vi "SCMP - Main Program.vi"() -> ()   [LabVIEW 2014]
doc: "Goodrich Exposure Range: .05microseconds to 798.9ms\n\nLow Gain (110e-/ADU)\nHigh Gain (6.5 e-/ADU)\n\nGA1280J Trigger Modes\n0 : Internally triggered; Internally timed\n1 : Externally triggered; Internally timed\n2 : Externally triggered; Externally timed\n3 : Externally gated; Internally timed\n\nFor list of camera commands\nsee Appendix A in the manual\n\n\nUse this template to build a standard state machine design pattern. Each state executes code and determines which state to transition to. Contrast this design pattern with the User Interface Event Handler pattern, in which code executes in response to user actions. Contrast this design pattern also with the Queued Message Handler pattern, in which each message handling code can queue zero or more new messages.\nNote: This template does not contain the most recent programming guidelines recommended by National Instruments. For a complete, project-based implementation of the Standard State Machine pattern, use the Create Project dialog box instead of this template."
uses:
  Controls/Main Program States.ctl
  <vilib>/Utility/error.llb/DialogType.ctl
  Controls/SCD - Calibration Optics Filter Wheel.ctl
  Controls/SCD - EDT - Emission Line Filter Wheel.ctl
  COMP/CoMP-S Controls/Emission Line Filter Wheel.ctl
  COMP/CoMP-S Controls/Polarization Optics Filter Wheel.ctl
  Controls/Global demo.vi
  C:/Users/mhutar/Documents/miro/lv_workdir github/SCMP/LabVIEW/COMP/Watlow EZ-ZONE/Public/Watbus.dll
  LabVIEW/COMP/Watlow EZ-ZONE/Public/Watbus.dll
  Controls/SCD - FITS Cluster.ctl
  AISAS/Controls/focus.ctl
  AISAS/Controls/Diffuser.ctl
  AISAS/Mech/AISAS Mech.lvclass
  Controls/peripherals.ctl
  Controls/Cbk Data type.ctl
  Controls/Cookbook.ctl
  Controls/beaning.ctl
  LabVIEW/Camera/Andor Neo Info.ctl
  PI/PI Control.ctl
panel:
  out "Instrument":string
  out "Main Loop":bool
  out "Log Loop":bool
  out "Program":bool
  out "Version":string
  in  "AOI Width 2":i64=2560
  in  "AOI Height 2":i64=2160
  in  "Observer":string="Observer"
  in  "Comment":string="Test"
  out "Latest Actions":string="\r"
  out "cbk name":string="automated_find_focus_656.cbk"
  out "Last Error":errorcluster={"status"=TRUE, "code"=0, "source"=""}
  in  "Tab Control":T1(tab)
  in  "PI cam3 (mm)":T2 min=0.1 max=27.0 step=0.1 format="%.1f"
  in  "PI cam2 (mm)":T2 min=0.1 max=31.0 step=0.1 format="%.1f"
  in  "Calibration Optics":T3
  in  "Occulter size":dbl format="%.2f"
  in  "Focus":T4 min=15.0 max=155.0 format="%.2f"
  in  "Andover Filter Wheel":T5
  in  "Calibration Wheel":T6
  in  "Binning":T7
  in  "Save Data to FITS? (F)":bool
  out "Histogram Graph":T8(graph)
  in  "Snap Images":bool
  in  "Live Preview (Andor)":bool
  out "Image":u16[][](graph)
  in  "Exposure (s)":dbl=0.02 min=1e-05 max=10.0 step=0.001 format="%_3p"
  out "Timestamp":timestamp=timestamp(3507746192.5616717 s since 1904-01-01)
  in  "PI cam1 (mm)":T2 min=0.1 max=29.0 step=0.1 format="%.1f"
  out "Snapshot FITS File Path":path
  in  "Emission Line Filters":T9
  in  "Set Filter Wheels":bool
  out "Mean ADU":u32=7788 format="%.1f"
  out "FITS Header":T10={"Wavelength (nm)"=530.15, "Exposure (s)"=0.05, "Tuning Delay (ms)"=1000.0, "Beam Type (-1/1)"=1.0, "Tuning Voltages"=[1.111, 2.222, 3.333, 4.444], "Observer"="observer", "Light Shapping Diffuser"=enum."In Beam", "Comment"="", "Data Type"=9, "Mod Cycles"=0, "SCD Calibration Optics"=enum."1 - Polarizer @0, I+Q", "SCD Emission Line Filter"=enum."1-557.6nm", "Cookbook"="", "COMP-S Calibration Wheel"=enum."Dark", "COMP-S Andover Filter Wheel"=enum."530.3nm/HWB 0.34nm (Fe XIV)", "FOV Rotation (deg)"=66.0, "Objective Lens Position (mm)"=0.0, "Occulter size"=0.0, "Time End"=timestamp(3382374145.421875 s since 1904-01-01), "Acc Exposure (s)"=0.0, "Time Stamp Array"=[], "Camera Serial Number"=[], "Camera Temp"=[], "Camera PI (mm)"=[], "Time Start"=timestamp(3382374145.421875 s since 1904-01-01), "Peripherals"={"ILX controler"=FALSE, "Zone temperatures"=FALSE, "Andor"=FALSE, "Andor 2"=FALSE, "PI Stage"=FALSE, "AISAS mechanisms"=FALSE, "AISAS Mech.lvclass"=refnum, "Zone temp ref"=variant}} {"Camera PI (mm)" format="%_3g"; "Acc Exposure (s)" format="%^.3g"; "Occulter size" format="%.2f"; "Objective Lens Position (mm)" min=15.0 max=155.0 format="%.2f"; "FOV Rotation (deg)" format="%.1f"; "Data Type" items=["LIVE", "DARK", "FLAT", "CALI", "OBSE", "ABSO", "AURE", "TARG", "OBJE", "HOLE", "OREX", "THRO", "CHIP"]; "Exposure (s)" format="%^.3g"; "Wavelength (nm)" format="%_6g"}
  out "Image Sharpness":dbl format="%.2f"
  in  "Diffuser":T11=enum."In Beam"
  in  "Rotation [deg]":dbl format="%.1f"
  in  "Move AISAS Mechanisms":bool
  in  "Motors":bool=TRUE
  out "Andor Neo":T13[](array[typedef]) {"Exposure (s)" format="%^.3g"; "Time at Synch" format="%<%H:%M:%S>T"; "Interframe Time" format="%#_3g"; "Frame Readout Time" format="%_3g"; "Row Readout Time" format="%_3g"}
  in  "Save Data to FITS?":bool=TRUE
  out "Cookbook":T15=[{"Data Type"=enum."SET EXPOSURE", "Arg 1"=200.0, "Arg 2"=999.0, "Arg 3"=path "C:/CoMP-S_Observer_cbks_rcps/mhutar/exposure-200ms.rcp", "Comments"=""}, {"Data Type"=enum."ACQUIRE DATA", "Arg 1"=1.0, "Arg 2"=1.0, "Arg 3"=path "C:/CoMP-S_Observer_cbks_rcps/mhutar/scan_530_3.rcp", "Comments"=""}]
  out "FITS Path from Last Recipe Acquiring Data":path
  in  "Load Cookbook":bool
  in  "Run Cookbook":bool
  out "# of Recipes":i16=2
  out "Selected Cookbook":path
  out "Recipe Files":string[](array[string])
  in  "FPS":dbl=10.0 min=0.1 max=49.0 step=1.0 format="%.1g"
  out "Continually Read Log File":string="20160903-07:42:55 Live Preview Images\n20160903-07:44:38 Program Terminated\n20160903-07:45:16 Program Started\n20160903-07:45:18 Snap Single Image\n20160903-07:45:27 Live Preview Images\n20160903-07:46:17 Calibration & Filter wheel position:\t8\t5\n20160903-07:46:35 Live Preview Images\n20160903-07:50:39 Live Preview Images\n20160903-07:51:54 Camera Moved to Positon:-18.00\n20160903-07:51:55 Snap Single Image\n20160903-07:52:37 Loaded Cookbook\tfind_focus_656.cbk\n20160903-07:53:52 Run Cookbook\tfind_focus_656.cbk\n20160903-07:53:52 Recipe#0-exposure-20ms.rcp\n20160903-07:53:52 Recipe#1-fw-656.rcp\n20160903-07:53:54 Recipe#2-cal-open.rcp\n20160903-07:53:56 Recipe#3-move-absolute-neg19.rcp\n20160903-07:53:56 Recipe#4-take_656_focus_image.rcp\n20160903-07:54:02 Recipe#5-move-relative-neg0pt25.rcp\n20160903-07:55:56 Program Started\n20160903-07:56:02 Camera Moved to Positon:-18.00\n20160903-07:56:03 Snap Single Image\n20160903-07:56:35 Camera Moved to Positon:-19.00\n20160903-07:56:37 Snap Single Image\n20160903-07:56:58 Camera Moved to Positon:-20.00\n20160903-07:57:02 Snap Single Image\n20160903-07:57:20 Camera Moved to Positon:-21.00\n20160903-07:57:23 Snap Single Image\n20160903-07:57:36 Camera Moved to Positon:-22.00\n20160903-07:57:37 Snap Single Image\n20160903-07:57:53 Camera Moved to Positon:-25.00\n20160903-07:57:57 Snap Single Image\n20160903-07:58:13 Camera Moved to Positon:-30.00\n20160903-07:58:17 Snap Single Image\n20160903-07:58:43 Camera Moved to Positon:-18.00\n20160903-07:58:44 Snap Single Image\n20160903-07:58:58 Camera Moved to Positon:-17.00\n20160903-07:59:00 Snap Single Image\n20160903-08:00:39 Calibration & Filter wheel position:\t7\t6\n20160903-08:00:48 Snap Single Image\n20160903-08:01:42 Camera Moved to Positon:-65.00\n20160903-08:01:47 Snap Single Image\n20160903-08:02:07 Camera Moved to Positon:-70.00\n20160903-08:02:10 Snap Single Image\n20160903-08:02:51 Camera Moved to Positon:-75.00\n20160903-08:02:53 Snap Single Image\n20160903-08:03:25 Calibration & Filter wheel position:\t7\t7\n20160903-08:03:37 Snap Single Image\n20160903-08:03:55 Camera Moved to Positon:-76.00\n20160903-08:04:01 Snap Single Image\n20160903-08:04:13 Camera Moved to Positon:-77.00\n20160903-08:04:14 Snap Single Image\n20160903-08:04:24 Camera Moved to Positon:-78.00\n20160903-08:04:26 Snap Single Image\n20160903-08:04:38 Camera Moved to Positon:-79.00\n20160903-08:04:39 Snap Single Image\n20160903-08:04:50 Camera Moved to Positon:-83.00\n20160903-08:04:52 Snap Single Image\n20160903-08:05:10 Camera Moved to Positon:-73.00\n20160903-08:05:11 Snap Single Image\n20160903-08:05:22 Camera Moved to Positon:-71.00\n20160903-08:05:24 Snap Single Image\n20160903-08:05:34 Camera Moved to Positon:-69.00\n20160903-08:05:35 Snap Single Image\n20160903-08:05:47 Camera Moved to Positon:-67.00\n20160903-08:05:48 Snap Single Image\n20160903-08:06:13 Calibration & Filter wheel position:\t7\t8\n20160903-08:07:06 Snap Single Image\n20160903-08:07:17 Camera Moved to Positon:-69.00\n20160903-08:07:18 Snap Single Image\n20160903-08:07:28 Camera Moved to Positon:-71.00\n20160903-08:07:30 Snap Single Image\n20160903-08:07:40 Camera Moved to Positon:-73.00\n20160903-08:07:43 Snap Single Image\n20160903-08:07:53 Camera Moved to Positon:-75.00\n20160903-08:07:55 Snap Single Image\n20160903-08:08:04 Camera Moved to Positon:-77.00\n20160903-08:08:06 Snap Single Image\n20160903-08:08:17 Camera Moved to Positon:-79.00\n20160903-08:08:28 Snap Single Image\n20160903-08:08:43 Camera Moved to Positon:-81.00\n20160903-08:08:46 Snap Single Image\n20160903-08:09:05 Calibration & Filter wheel position:\t7\t9\n20160903-08:09:48 Camera Moved to Positon:-100.00\n20160903-08:09:50 Snap Single Image\n20160903-08:10:09 Snap Single Image\n20160903-08:10:26 Camera Moved to Positon:-100.00\n20160903-08:10:35 Camera Moved to Positon:-100.00\n20160903-08:10:37 Snap Single Image\n20160903-08:10:54 Camera Moved to Positon:-100.00\n20160903-08:10:59 Program Terminated\n20160903-08:12:25 Program Started\n20160903-08:12:33 Camera Moved to Positon:-100.00\n20160903-08:12:38 Program Terminated\n20160903-08:13:25 Program Started\n20160903-08:13:30 Camera Moved to Positon:-100.00\n20160903-08:13:37 Program Terminated\n20160903-08:14:12 Program Started\n20160903-08:14:19 Camera Moved to Positon:-100.00\n20160903-08:14:22 Snap Single Image\n20160903-08:14:37 Calibration & Filter wheel position:\t7\t9\n20160903-08:14:45 Snap Single Image\n20160903-08:14:56 Camera Moved to Positon:-105.00\n20160903-08:14:57 Snap Single Image\n20160903-08:15:10 Camera Moved to Positon:-110.00\n20160903-08:15:11 Snap Single Image\n20160903-08:15:23 Camera Moved to Positon:-115.00\n20160903-08:15:27 Snap Single Image\n20160903-08:15:39 Camera Moved to Positon:-120.00\n20160903-08:15:40 Snap Single Image\n20160903-08:15:59 Snap Single Image\n20160903-08:16:10 Camera Moved to Positon:-115.00\n20160903-08:16:11 Snap Single Image\n20160903-08:16:21 Camera Moved to Positon:-110.00\n20160903-08:16:22 Snap Single Image\n20160903-08:16:33 Camera Moved to Positon:-105.00\n20160903-08:16:36 Snap Single Image\n20160903-08:16:49 Camera Moved to Positon:-100.00\n20160903-08:16:51 Snap Single Image\n20160903-08:17:03 Camera Moved to Positon:-95.00\n20160903-08:17:05 Snap Single Image\n20160903-08:17:16 Camera Moved to Positon:-90.00\n20160903-08:17:18 Snap Single Image\n20160903-08:17:46 Camera Moved to Positon:-85.00\n20160903-08:17:49 Snap Single Image\n20160903-08:18:00 Camera Moved to Positon:-80.00\n20160903-08:18:02 Snap Single Image\n20160903-08:18:40 Calibration & Filter wheel position:\t7\t4\n20160903-08:18:59 Camera Moved to Positon:-20.00\n20160903-08:19:11 Snap Single Image\n20160903-08:19:23 Camera Moved to Positon:-18.00\n20160903-08:19:25 Snap Single Image\n20160903-08:19:38 Camera Moved to Positon:-22.00\n20160903-08:19:39 Snap Single Image\n20160903-08:19:51 Camera Moved to Positon:-24.00\n20160903-08:19:52 Snap Single Image\n20160903-08:20:04 Calibration & Filter wheel position:\t7\t3\n20160903-08:20:11 Snap Single Image\n20160903-08:20:22 Camera Moved to Positon:-18.00\n20160903-08:20:24 Snap Single Image\n20160903-08:20:39 Camera Moved to Positon:-16.00\n20160903-08:20:40 Snap Single Image\n20160903-08:20:53 Camera Moved to Positon:-14.00\n20160903-08:20:56 Snap Single Image\n20160903-08:21:06 Camera Moved to Positon:-12.00\n20160903-08:21:07 Snap Single Image\n20160903-08:21:16 Camera Moved to Positon:-10.00\n20160903-08:21:24 Snap Single Image\n20160903-08:21:34 Camera Moved to Positon: -8.00\n20160903-08:21:36 Snap Single Image\n20160903-08:22:12 Camera Moved to Positon: -6.00\n20160903-08:22:21 Snap Single Image\n20160903-08:23:09 Calibration & Filter wheel position:\t7\t1\n20160903-08:23:17 Snap Single Image\n20160903-08:23:27 Camera Moved to Positon: -4.00\n20160903-08:23:29 Snap Single Image\n20160903-08:23:37 Camera Moved to Positon: -2.00\n20160903-08:23:38 Snap Single Image\n20160903-08:23:47 Camera Moved to Positon:  0.00\n20160903-08:23:50 Snap Single Image\n20160903-08:26:00 Camera Moved to Positon:-18.00\n20160903-08:26:44 Program Started\n20160903-08:26:59 Camera Moved to Positon:-18.00\n20160903-08:27:05 Loaded Cookbook\tfind_focus_656.cbk\n20160903-08:27:12 Run Cookbook\tfind_focus_656.cbk\n20160903-08:27:12 Recipe#0-exposure-20ms.rcp\n20160903-08:27:12 Recipe#1-fw-656.rcp\n20160903-08:27:14 Recipe#2-cal-open.rcp\n20160903-08:27:16 Recipe#3-take_656_focus_image.rcp\n20160903-08:29:11 Camera Moved to Positon:-19.00\n20160903-08:29:17 Run Cookbook\tfind_focus_656.cbk\n20160903-08:29:17 Recipe#0-exposure-20ms.rcp\n20160903-08:29:17 Recipe#1-fw-656.rcp\n20160903-08:29:19 Recipe#2-cal-open.rcp\n20160903-08:29:21 Recipe#3-take_656_focus_image.rcp\n20160903-08:29:59 Camera Moved to Positon:-20.00\n20160903-08:30:03 Run Cookbook\tfind_focus_656.cbk\n20160903-08:30:03 Recipe#0-exposure-20ms.rcp\n20160903-08:30:03 Recipe#1-fw-656.rcp\n20160903-08:30:05 Recipe#2-cal-open.rcp\n20160903-08:30:07 Recipe#3-take_656_focus_image.rcp\n20160903-08:30:28 Camera Moved to Positon:-21.00\n20160903-08:30:32 Run Cookbook\tfind_focus_656.cbk\n20160903-08:30:32 Recipe#0-exposure-20ms.rcp\n20160903-08:30:32 Recipe#1-fw-656.rcp\n20160903-08:30:34 Recipe#2-cal-open.rcp\n20160903-08:30:36 Recipe#3-take_656_focus_image.rcp\n20160903-08:31:03 Camera Moved to Positon:-22.00\n20160903-08:31:06 Run Cookbook\tfind_focus_656.cbk\n20160903-08:31:06 Recipe#0-exposure-20ms.rcp\n20160903-08:31:06 Recipe#1-fw-656.rcp\n20160903-08:31:08 Recipe#2-cal-open.rcp\n20160903-08:31:10 Recipe#3-take_656_focus_image.rcp\n20160903-08:31:33 Camera Moved to Positon:-23.00\n20160903-08:31:38 Run Cookbook\tfind_focus_656.cbk\n20160903-08:31:38 Recipe#0-exposure-20ms.rcp\n20160903-08:31:38 Recipe#1-fw-656.rcp\n20160903-08:31:40 Recipe#2-cal-open.rcp\n20160903-08:31:42 Recipe#3-take_656_focus_image.rcp\n20160903-08:32:05 Camera Moved to Positon:-24.00\n20160903-08:32:08 Run Cookbook\tfind_focus_656.cbk\n20160903-08:32:08 Recipe#0-exposure-20ms.rcp\n20160903-08:32:08 Recipe#1-fw-656.rcp\n20160903-08:32:10 Recipe#2-cal-open.rcp\n20160903-08:32:12 Recipe#3-take_656_focus_image.rcp\n20160903-08:32:35 Camera Moved to Positon:-25.00\n20160903-08:32:40 Run Cookbook\tfind_focus_656.cbk\n20160903-08:32:40 Recipe#0-exposure-20ms.rcp\n20160903-08:32:40 Recipe#1-fw-656.rcp\n20160903-08:32:42 Recipe#2-cal-open.rcp\n20160903-08:32:44 Recipe#3-take_656_focus_image.rcp\n20160903-08:33:03 Camera Moved to Positon:-26.00\n20160903-08:33:07 Run Cookbook\tfind_focus_656.cbk\n20160903-08:33:07 Recipe#0-exposure-20ms.rcp\n20160903-08:33:07 Recipe#1-fw-656.rcp\n20160903-08:33:09 Recipe#2-cal-open.rcp\n20160903-08:33:11 Recipe#3-take_656_focus_image.rcp\n20160903-08:33:32 Camera Moved to Positon:-27.00\n20160903-08:33:34 Run Cookbook\tfind_focus_656.cbk\n20160903-08:33:34 Recipe#0-exposure-20ms.rcp\n20160903-08:33:34 Recipe#1-fw-656.rcp\n20160903-08:33:36 Recipe#2-cal-open.rcp\n20160903-08:33:38 Recipe#3-take_656_focus_image.rcp\n20160903-08:34:01 Camera Moved to Positon:-28.00\n20160903-08:34:05 Run Cookbook\tfind_focus_656.cbk\n20160903-08:34:05 Recipe#0-exposure-20ms.rcp\n20160903-08:34:05 Recipe#1-fw-656.rcp\n20160903-08:34:07 Recipe#2-cal-open.rcp\n20160903-08:34:09 Recipe#3-take_656_focus_image.rcp\n20160903-08:36:44 Camera Moved to Positon:-85.00\n20160903-08:36:51 Loaded Cookbook\tfind_focus_1083.cbk\n20160903-08:37:11 Loaded Cookbook\tfind_focus_1083.cbk\n20160903-08:37:20 Run Cookbook\tfind_focus_1083.cbk\n20160903-08:37:20 Recipe#0-exposure-120ms.rcp\n20160903-08:37:20 Recipe#1-fw-1083.rcp\n20160903-08:37:22 Recipe#2-cal-open.rcp\n20160903-08:37:23 Recipe#3-take_1083_focus_image.rcp\n20160903-08:38:05 Camera Moved to Positon:-86.00\n20160903-08:38:11 Run Cookbook\tfind_focus_1083.cbk\n20160903-08:38:11 Recipe#0-exposure-120ms.rcp\n20160903-08:38:11 Recipe#1-fw-1083.rcp\n20160903-08:38:13 Recipe#2-cal-open.rcp\n20160903-08:38:15 Recipe#3-take_1083_focus_image.rcp\n20160903-08:38:39 Camera Moved to Positon:-87.00\n20160903-08:38:43 Run Cookbook\tfind_focus_1083.cbk\n20160903-08:38:43 Recipe#0-exposure-120ms.rcp\n20160903-08:38:43 Recipe#1-fw-1083.rcp\n20160903-08:38:45 Recipe#2-cal-open.rcp\n20160903-08:38:47 Recipe#3-take_1083_focus_image.rcp\n20160903-08:39:05 Camera Moved to Positon:-88.00\n20160903-08:39:09 Run Cookbook\tfind_focus_1083.cbk\n20160903-08:39:10 Recipe#0-exposure-120ms.rcp\n20160903-08:39:10 Recipe#1-fw-1083.rcp\n20160903-08:39:12 Recipe#2-cal-open.rcp\n20160903-08:39:13 Recipe#3-take_1083_focus_image.rcp\n20160903-08:43:45 Snap Single Image\n20160903-08:43:56 Run Cookbook\tfind_focus_1083.cbk\n20160903-08:43:56 Recipe#0-exposure-120ms.rcp\n20160903-08:43:56 Recipe#1-fw-1083.rcp\n20160903-08:43:58 Recipe#2-cal-open.rcp\n20160903-08:44:00 Recipe#3-take_1083_focus_image.rcp\n20160903-08:44:24 Camera Moved to Positon:-90.00\n20160903-08:44:32 Camera Moved to Positon:-89.00\n20160903-08:44:36 Run Cookbook\tfind_focus_1083.cbk\n20160903-08:44:36 Recipe#0-exposure-120ms.rcp\n20160903-08:44:36 Recipe#1-fw-1083.rcp\n20160903-08:44:38 Recipe#2-cal-open.rcp\n20160903-08:44:40 Recipe#3-take_1083_focus_image.rcp\n20160903-08:45:03 Camera Moved to Positon:-90.00\n20160903-08:45:11 Run Cookbook\tfind_focus_1083.cbk\n20160903-08:45:12 Recipe#0-exposure-120ms.rcp\n20160903-08:45:12 Recipe#1-fw-1083.rcp\n20160903-08:45:14 Recipe#2-cal-open.rcp\n20160903-08:45:15 Recipe#3-take_1083_focus_image.rcp\n20160903-08:45:38 Camera Moved to Positon:-91.00\n20160903-08:45:41 Run Cookbook\tfind_focus_1083.cbk\n20160903-08:45:41 Recipe#0-exposure-120ms.rcp\n20160903-08:45:42 Recipe#1-fw-1083.rcp\n20160903-08:45:43 Recipe#2-cal-open.rcp\n20160903-08:45:45 Recipe#3-take_1083_focus_image.rcp\n20160903-08:46:07 Camera Moved to Positon:-92.00\n20160903-08:46:12 Run Cookbook\tfind_focus_1083.cbk\n20160903-08:46:12 Recipe#0-exposure-120ms.rcp\n20160903-08:46:12 Recipe#1-fw-1083.rcp\n20160903-08:46:14 Recipe#2-cal-open.rcp\n20160903-08:46:16 Recipe#3-take_1083_focus_image.rcp\n20160903-08:46:53 Camera Moved to Positon:-93.00\n20160903-08:46:56 Run Cookbook\tfind_focus_1083.cbk\n20160903-08:46:56 Recipe#0-exposure-120ms.rcp\n20160903-08:46:56 Recipe#1-fw-1083.rcp\n20160903-08:46:58 Recipe#2-cal-open.rcp\n20160903-08:47:00 Recipe#3-take_1083_focus_image.rcp\n20160903-08:48:13 Calibration & Filter wheel position:\t7\t3\n20160903-08:51:11 Camera Moved to Positon:-10.00\n20160903-08:51:19 Camera Moved to Positon: -5.00\n20160903-08:51:20 Live Preview Images\n20160903-08:51:43 Loaded Cookbook\tfind_focus_589.cbk\n20160903-08:52:08 Loaded Cookbook\tfocus-656.cbk\n20160903-08:52:09 Run Cookbook\tfocus-656.cbk\n20160903-08:52:09 Recipe#0-fw-656.rcp\n20160903-08:52:11 Recipe#1-cal-clear.rcp\n20160903-08:52:13 Recipe#2-exposure-200ms.rcp\n20160903-08:52:13 Recipe#3-focus-656.rcp\n20160903-08:52:24 Program Started\n20160903-08:52:33 Loaded Cookbook\tfocus-656.cbk\n20160903-08:52:40 Camera Moved to Positon: -5.00\n20160903-08:52:46 Loaded Cookbook\tfind_focus_589.cbk\n20160903-08:52:48 Run Cookbook\tfind_focus_589.cbk\n20160903-08:52:48 Recipe#0-exposure-20ms.rcp\n20160903-08:52:48 Recipe#1-fw-589.rcp\n20160903-08:52:50 Recipe#2-cal-open.rcp\n20160903-08:52:52 Recipe#3-take_589_focus_image.rcp\n20160903-08:54:55 Run Cookbook\tfind_focus_589.cbk\n20160903-08:54:55 Recipe#0-exposure-20ms.rcp\n20160903-08:54:56 Recipe#1-fw-589.rcp\n20160903-08:54:57 Recipe#2-cal-open.rcp\n20160903-08:54:59 Recipe#3-take_589_focus_image.rcp\n20160903-08:55:19 Live Preview Images\n20160903-08:56:01 Camera Moved to Positon: -6.00\n20160903-08:56:04 Run Cookbook\tfind_focus_589.cbk\n20160903-08:56:04 Recipe#0-exposure-20ms.rcp\n20160903-08:56:04 Recipe#1-fw-589.rcp\n20160903-08:56:06 Recipe#2-cal-open.rcp\n20160903-08:56:08 Recipe#3-take_589_focus_image.rcp\n20160903-08:56:40 Camera Moved to Positon: -7.00\n20160903-08:58:30 Run Cookbook\tfind_focus_589.cbk\n20160903-08:58:30 Recipe#0-exposure-20ms.rcp\n20160903-08:58:30 Recipe#1-fw-589.rcp\n20160903-08:58:32 Recipe#2-cal-open.rcp\n20160903-08:58:34 Recipe#3-take_589_focus_image.rcp\n20160903-08:59:22 Camera Moved to Positon: -8.00\n20160903-09:14:18 Program Terminated\n20160903-09:40:55 Program Started\n20160903-09:44:03 Loaded Cookbook\tautomated_find_focus_656.cbk\n20160903-09:44:43 Loaded Cookbook\tautomated_find_focus_656.cbk\n20160903-09:44:57 Run Cookbook\tautomated_find_focus_656.cbk\n20160903-09:44:57 Recipe#0-exposure-20ms.rcp\n20160903-09:44:57 Recipe#1-fw-656.rcp\n20160903-09:44:59 Recipe#2-cal-open.rcp\n20160903-09:45:01 Recipe#3-move-absolute-neg15.rcp\n20160903-09:45:02 Recipe#4-take_656_focus_image.rcp\n20160903-09:45:16 Recipe#5-move-relative-neg0pt25.rcp\n20160903-09:45:17 Recipe#6-take_656_focus_image.rcp\n20160903-09:45:31 Recipe#7-move-relative-neg0pt25.rcp\n20160903-09:45:32 Recipe#8-take_656_focus_image.rcp\n20160903-09:45:46 Recipe#9-move-relative-neg0pt25.rcp\n20160903-09:45:47 Recipe#10-take_656_focus_image.rcp\n20160903-09:46:01 Recipe#11-move-relative-neg0pt25.rcp\n20160903-09:46:02 Recipe#12-take_656_focus_image.rcp\n20160903-09:46:17 Recipe#13-move-relative-neg0pt25.rcp\n20160903-09:46:18 Recipe#14-take_656_focus_image.rcp\n20160903-09:46:32 Recipe#15-move-relative-neg0pt25.rcp\n20160903-09:46:33 Recipe#16-take_656_focus_image.rcp\n20160903-09:46:47 Recipe#17-move-relative-neg0pt25.rcp\n20160903-09:46:48 Recipe#18-take_656_focus_image.rcp\n20160903-09:47:02 Recipe#19-move-relative-neg0pt25.rcp\n20160903-09:47:03 Recipe#20-take_656_focus_image.rcp\n20160903-09:47:17 Recipe#21-move-relative-neg0pt25.rcp\n20160903-09:47:17 Recipe#22-take_656_focus_image.rcp\n20160903-09:47:32 Recipe#23-move-relative-neg0pt25.rcp\n20160903-09:47:32 Recipe#24-take_656_focus_image.rcp\n20160903-09:47:46 Recipe#25-move-relative-neg0pt25.rcp\n20160903-09:47:47 Recipe#26-take_656_focus_image.rcp\n20160903-09:48:02 Recipe#27-move-relative-neg0pt25.rcp\n20160903-09:48:03 Recipe#28-take_656_focus_image.rcp\n20160903-09:48:17 Recipe#29-move-relative-neg0pt25.rcp\n20160903-09:48:17 Recipe#30-take_656_focus_image.rcp\n20160903-09:48:32 Recipe#31-move-relative-neg0pt25.rcp\n20160903-09:48:33 Recipe#32-take_656_focus_image.rcp\n20160903-09:48:49 Recipe#33-move-relative-neg0pt25.rcp\n20160903-09:48:49 Recipe#34-take_656_focus_image.rcp\n20160903-09:49:05 Recipe#35-move-relative-neg0pt25.rcp\n20160903-09:49:06 Recipe#36-take_656_focus_image.rcp\n20160903-09:49:23 Recipe#37-move-relative-neg0pt25.rcp\n20160903-09:49:24 Recipe#38-take_656_focus_image.rcp\n20160903-09:49:41 Recipe#39-move-relative-neg0pt25.rcp\n20160903-09:49:42 Recipe#40-take_656_focus_image.rcp\n20160903-09:50:01 Recipe#41-move-relative-neg0pt25.rcp\n20160903-09:50:01 Recipe#42-take_656_focus_image.rcp\n20160903-09:50:20 Recipe#43-move-relative-neg0pt25.rcp\n20160903-09:50:21 Recipe#44-take_656_focus_image.rcp\n20160903-09:54:36 Loaded Cookbook\tautomated_find_focus_656.cbk\n20160903-09:54:47 Loaded Cookbook\tautomated_find_focus_656.cbk\n20160903-09:55:40 Loaded Cookbook\tautomated_find_focus_656.cbk\n20160903-09:55:54 Run Cookbook\tautomated_find_focus_656.cbk\n20160903-09:55:54 Recipe#0-exposure-40ms.rcp\n20160903-09:55:54 Recipe#1-fw-656.rcp\n20160903-09:55:56 Recipe#2-cal-open.rcp\n20160903-09:55:58 Recipe#3-move-absolute-neg15.rcp\n20160903-09:55:59 Recipe#4-take_656_focus_image.rcp\n20160903-09:56:06 Recipe#5-move-relative-neg0pt5.rcp\n20160903-09:56:07 Recipe#6-take_656_focus_image.rcp\n20160903-09:56:14 Recipe#7-move-relative-neg0pt5.rcp\n20160903-09:56:15 Recipe#8-take_656_focus_image.rcp\n20160903-09:56:22 Recipe#9-move-relative-neg0pt5.rcp\n20160903-09:56:22 Recipe#10-take_656_focus_image.rcp\n20160903-09:56:29 Recipe#11-move-relative-neg0pt5.rcp\n20160903-09:56:30 Recipe#12-take_656_focus_image.rcp\n20160903-09:56:37 Recipe#13-move-relative-neg0pt5.rcp\n20160903-09:56:38 Recipe#14-take_656_focus_image.rcp\n20160903-09:56:45 Recipe#15-move-relative-neg0pt5.rcp\n20160903-09:56:45 Recipe#16-take_656_focus_image.rcp\n20160903-09:56:52 Recipe#17-move-relative-neg0pt5.rcp\n20160903-09:56:53 Recipe#18-take_656_focus_image.rcp\n20160903-09:57:00 Recipe#19-move-relative-neg0pt5.rcp\n20160903-09:57:01 Recipe#20-take_656_focus_image.rcp\n20160903-09:57:08 Recipe#21-move-relative-neg0pt5.rcp\n20160903-09:57:09 Recipe#22-take_656_focus_image.rcp\n20160903-09:57:16 Recipe#23-move-relative-neg0pt5.rcp\n20160903-09:57:16 Recipe#24-take_656_focus_image.rcp\n20160903-09:57:23 Recipe#25-move-relative-neg0pt5.rcp\n20160903-09:57:24 Recipe#26-take_656_focus_image.rcp\n20160903-09:57:31 Recipe#27-move-relative-neg0pt5.rcp\n20160903-09:57:32 Recipe#28-take_656_focus_image.rcp\n20160903-09:57:39 Recipe#29-move-relative-neg0pt5.rcp\n20160903-09:57:40 Recipe#30-take_656_focus_image.rcp\n20160903-09:57:47 Recipe#31-move-relative-neg0pt5.rcp\n20160903-09:57:48 Recipe#32-take_656_focus_image.rcp\n20160903-09:57:55 Recipe#33-move-relative-neg0pt5.rcp\n20160903-09:57:56 Recipe#34-take_656_focus_image.rcp\n20160903-09:58:03 Recipe#35-move-relative-neg0pt5.rcp\n20160903-09:58:03 Recipe#36-take_656_focus_image.rcp\n20160903-09:58:10 Recipe#37-move-relative-neg0pt5.rcp\n20160903-09:58:11 Recipe#38-take_656_focus_image.rcp\n20160903-09:58:18 Recipe#39-move-relative-neg0pt5.rcp\n20160903-09:58:19 Recipe#40-take_656_focus_image.rcp\n20160903-09:58:26 Recipe#41-move-relative-neg0pt5.rcp\n20160903-09:58:27 Recipe#42-take_656_focus_image.rcp\n20160903-09:58:34 Recipe#43-move-relative-neg0pt5.rcp\n20160903-09:58:35 Recipe#44-take_656_focus_image.rcp\n20160903-10:46:33 Program Terminated\n20160903-12:25:32 Program Started\n20160903-12:26:22 Program Terminated\n20160903-12:45:45 Program Started\n20160903-12:45:56 Program Terminated\n20160903-12:49:12 Program Started\n20160903-12:49:15 Loaded Cookbook\tautomated_find_focus_656.cbk\n20160903-12:49:24 Run Cookbook\tautomated_find_focus_656.cbk\n20160903-12:49:25 Recipe#0-exposure-40ms.rcp\n20160903-12:49:25 Recipe#1-fw-656.rcp\n20160903-12:49:26 Recipe#2-cal-open.rcp\n20160903-12:49:28 Recipe#3-move-absolute-neg15.rcp\n20160903-12:49:29 Recipe#4-take_656_focus_image.rcp\n20160903-12:49:32 Recipe#5-move-relative-neg0pt5.rcp\n20160903-12:49:33 Recipe#6-take_656_focus_image.rcp\n20160903-12:49:36 Recipe#7-move-relative-neg0pt5.rcp\n20160903-12:49:36 Recipe#8-take_656_focus_image.rcp\n20160903-12:49:39 Recipe#9-move-relative-neg0pt5.rcp\n20160903-12:49:40 Recipe#10-take_656_focus_image.rcp\n20160903-12:49:43 Recipe#11-move-relative-neg0pt5.rcp\n20160903-12:49:43 Recipe#12-take_656_focus_image.rcp\n20160903-12:49:46 Recipe#13-move-relative-neg0pt5.rcp\n20160903-12:49:47 Recipe#14-take_656_focus_image.rcp\n20160903-12:49:49 Recipe#15-move-relative-neg0pt5.rcp\n20160903-12:49:50 Recipe#16-take_656_focus_image.rcp\n20160903-12:49:53 Recipe#17-move-relative-neg0pt5.rcp\n20160903-12:49:53 Recipe#18-take_656_focus_image.rcp\n20160903-12:49:56 Recipe#19-move-relative-neg0pt5.rcp\n20160903-12:49:57 Recipe#20-take_656_focus_image.rcp\n20160903-12:49:59 Recipe#21-move-relative-neg0pt5.rcp\n20160903-12:50:00 Recipe#22-take_656_focus_image.rcp\n20160903-12:50:03 Recipe#23-move-relative-neg0pt5.rcp\n20160903-12:50:04 Recipe#24-take_656_focus_image.rcp\n20160903-12:50:06 Recipe#25-move-relative-neg0pt5.rcp\n20160903-12:50:07 Recipe#26-take_656_focus_image.rcp\n20160903-12:50:10 Recipe#27-move-relative-neg0pt5.rcp\n20160903-12:50:10 Recipe#28-take_656_focus_image.rcp\n20160903-12:50:13 Recipe#29-move-relative-neg0pt5.rcp\n20160903-12:50:14 Recipe#30-take_656_focus_image.rcp\n20160903-12:50:16 Recipe#31-move-relative-neg0pt5.rcp\n20160903-12:50:17 Recipe#32-take_656_focus_image.rcp\n20160903-12:50:20 Recipe#33-move-relative-neg0pt5.rcp\n20160903-12:50:20 Recipe#34-take_656_focus_image.rcp\n20160903-12:50:23 Recipe#35-move-relative-neg0pt5.rcp\n20160903-12:50:24 Recipe#36-take_656_focus_image.rcp\n20160903-12:50:26 Recipe#37-move-relative-neg0pt5.rcp\n20160903-12:50:27 Recipe#38-take_656_focus_image.rcp\n20160903-12:50:30 Recipe#39-move-relative-neg0pt5.rcp\n20160903-12:50:31 Recipe#40-take_656_focus_image.rcp\n20160903-12:50:33 Recipe#41-move-relative-neg0pt5.rcp\n20160903-12:50:34 Recipe#42-take_656_focus_image.rcp\n20160903-12:50:37 Recipe#43-move-relative-neg0pt5.rcp\n20160903-12:50:37 Recipe#44-take_656_focus_image.rcp\n20160903-13:54:17 Program Terminated\n20160903-14:07:18 Program Started\n20160903-14:08:12 Program Terminated\n20160903-14:20:46 Program Started\n20160903-14:22:56 Program Terminated\n20160903-14:23:20 Program Started\n20160903-14:25:03 Program Terminated\n20160903-14:31:16 Program Started\n20160903-14:32:59 Program Terminated\n20160903-14:33:26 Program Started\n20160903-14:35:01 Program Terminated\n20160903-14:36:43 Program Started\n20160903-14:38:01 Program Terminated\n20160903-14:39:22 Program Started\n20160903-14:39:47 Program Terminated\n20160903-14:40:22 Program Started\n20160903-14:41:59 Program Terminated\n20160903-15:07:40 Program Started\n20160903-15:10:18 Program Terminated\n20160903-15:19:59 Program Started\n20160903-15:20:17 Program Terminated\n20160903-15:20:43 Program Started\n20160903-15:20:43 Program Terminated\n20160903-15:21:33 Program Started\n20160903-15:22:45 Program Terminated\n20160903-15:24:43 Program Started\n20160903-15:26:40 Program Terminated\n20160903-15:29:07 Program Started\n20160903-15:29:52 Loaded Cookbook\tautomated_find_focus_656.cbk\n20160903-15:30:08 Loaded Cookbook\tautomated_find_focus_656.cbk\n"
  out "max Cookbook Exposure [s]":dbl=200.0 format="%#_3p"
  out "Today's SCMP Log File":path
  out "Cookbook Comments":string
  in  "Mod/Seq":bool
  out "Camera 2 Temp [C}":dbl(graph)=-21.03
  in  "Log loop delay [s]":dbl=10.0
  in  "Enable Data Logging":bool=TRUE
  out "Today's SCMP Eng  File":path
  out "Air around \nprefilter wheel [C]":sgl(graph)
  out "Lyot Filter Temp [C]":dbl(graph)
  out "Air around Camera [C]":sgl(graph)
  out "Air around Lyot Filter [C]":dbl(graph)
  out "Data Logging Error":errorcluster={"status"=TRUE, "code"=0, "source"=""}
  out "Camera 1 Temp [C}":dbl(graph)=-21.03
  out "Main Loop Error":errorcluster={"status"=TRUE, "code"=0, "source"=""}
  in  "Stop":bool=TRUE
  # "Camera Settings"
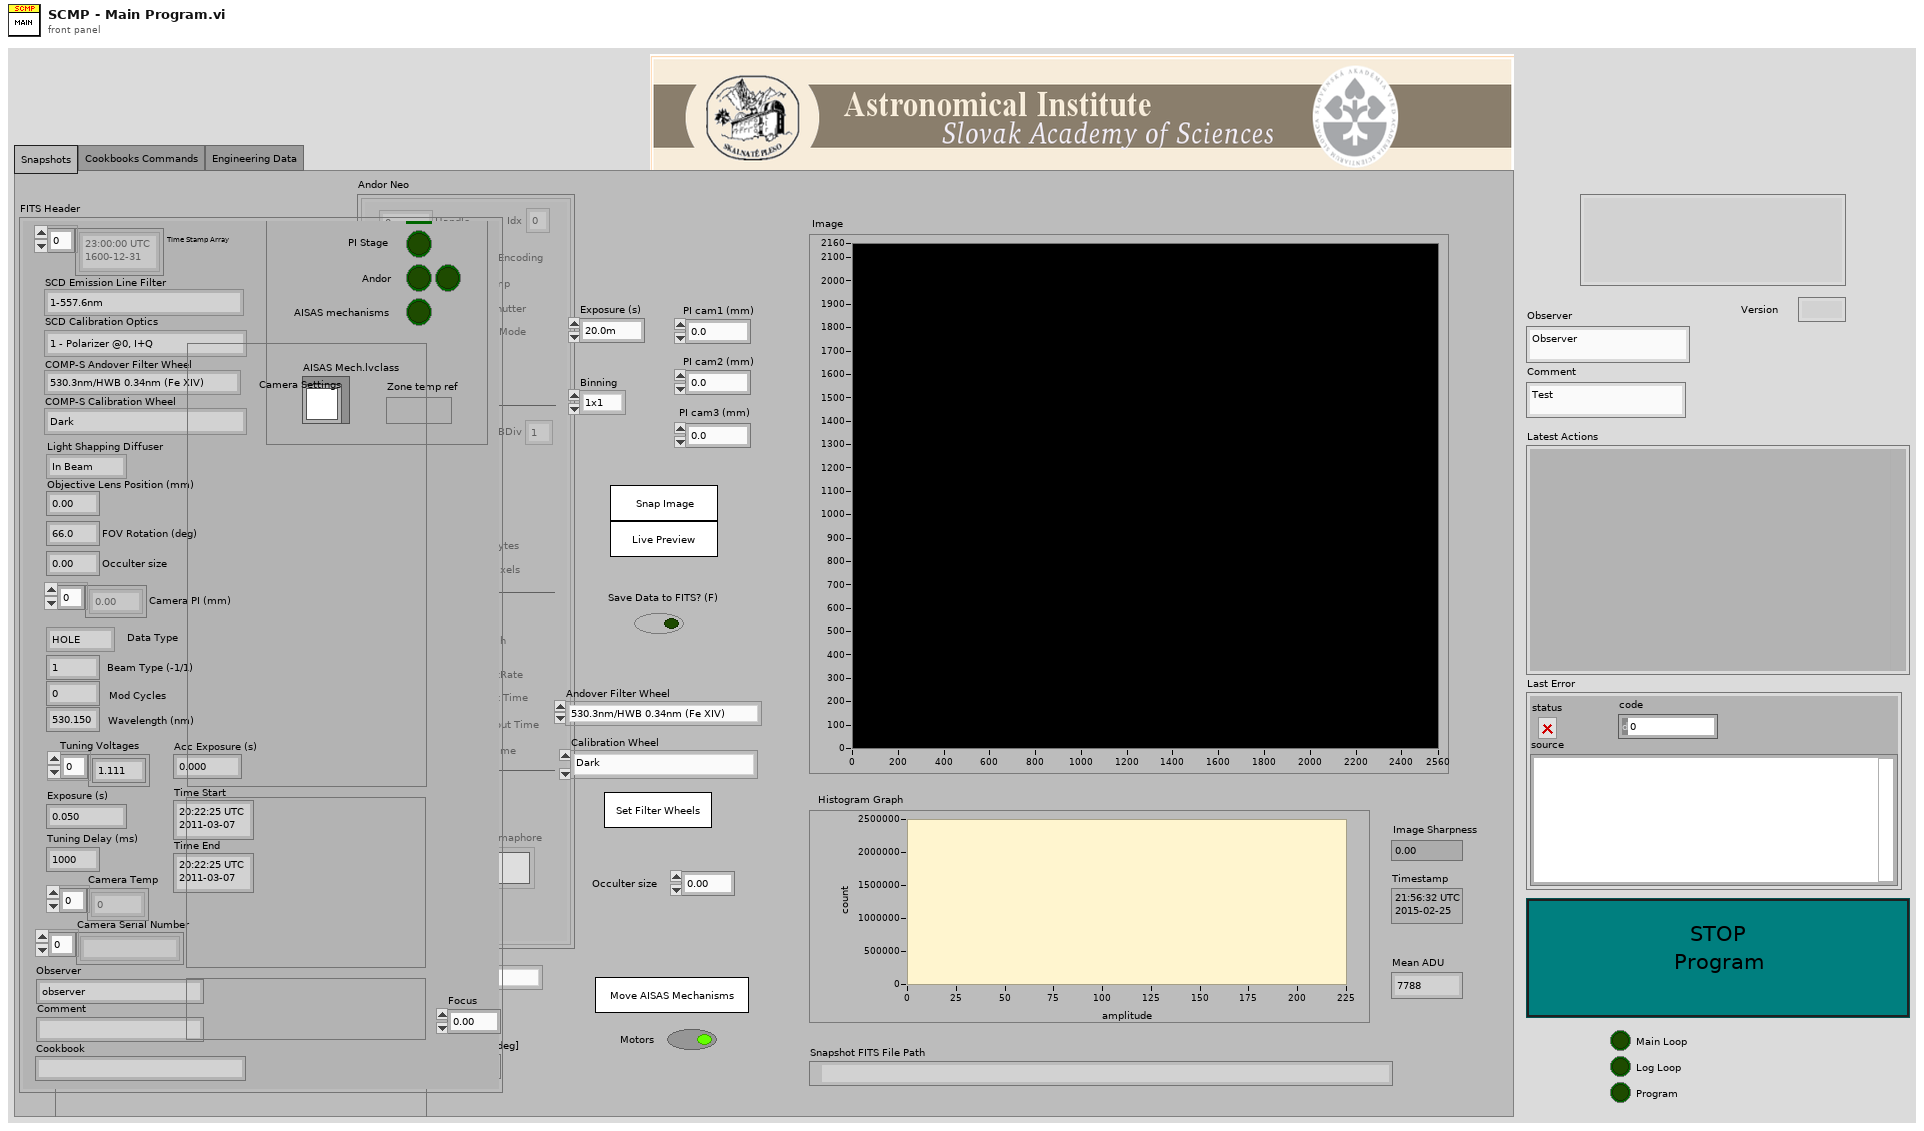
[diagram p1: front panel]
types:
  T1 = enum32{"Snapshots", "Cookbooks Commands", "Engineering Data"}
  T2 = typedef "PI Control.ctl" = dbl
  T3 = typedef "SCD - Calibration Optics Filter Wheel.ctl" = enum16{"1 - Polarizer @0, I+Q", "2 - Polarizer @90, I-Q", "3 - Polarizer @45, I+U", "4 - Polarizer @135, I-U", "5 - Polarizer @0, Retarder @45, I+V", "6 - Polarizer @0, Retarder @135, I-V", "7 - Dark", "8 - Clear", "9 - N/A"}
  T4 = typedef "focus.ctl" = dbl
  T5 = typedef "Emission Line Filter Wheel.ctl" = enum16{"530.3nm/HWB 0.34nm (Fe XIV)", "587.6nm/HBW 0.44nm (He I D3)", "637.5nm/HBW 0.53nm (Fe X)", "656.3nm/HBW 0.57nm (H-Alpha)", "789.2nm/HBW 0.85nm (Fe XI)", "854.2nm/HBW 1.01nm (Ca I)", "1074.7nm/HBW 2.34nm (Fe XIII)", "1079.8nm/HBW 1.64nm (Fe XIII)", "1083.0nm/HBW 1.66nm (He I)"}
  T6 = typedef "Polarization Optics Filter Wheel.ctl" = enum16{"Dark", "Clear", "Exchange Lens", "Polarizer @0, I+Q", "Polarizer @90, I-Q", "Polarizer @45, I+U", "Polarizer @135, I-U", "Polarizer @0, Retarder @45, I+V", "Polarizer @0, Retarder @135, I-V"}
  T7 = typedef "beaning.ctl" = enum16{"1x1", "2x2", "3x3", "4x4", "8x8"}
  T8 = cluster{"X Values":dbl[], "Histogram: h(x)":i32[]}[]
  T9 = typedef "SCD - EDT - Emission Line Filter Wheel.ctl" = enum16{"1-557.6nm", "2-587.6nm", "3-589.6nm", "4-630.2nm", "5-656.4nm", "6-849.8nm", "7-854.2nm", "8-866.2nm", "9-1083.0nm"}
  T10 = typedef "SCD - FITS Cluster.ctl" = cluster{"Wavelength (nm)":dbl, "Exposure (s)":dbl, "Tuning Delay (ms)":dbl, "Beam Type (-1/1)":dbl, "Tuning Voltages":dbl[], "Observer":string, "Light Shapping Diffuser":T11, "Comment":string, "Data Type":u16, "Mod Cycles":u16, "SCD Calibration Optics":T3, "SCD Emission Line Filter":T9, "Cookbook":string, "COMP-S Calibration Wheel":T6, "COMP-S Andover Filter Wheel":T5, "FOV Rotation (deg)":dbl, "Objective Lens Position (mm)":T4, "Occulter size":dbl, "Time End":timestamp, "Acc Exposure (s)":dbl, "Time Stamp Array":timestamp[], "Camera Serial Number":string[], "Camera Temp":dbl[], "Camera PI (mm)":dbl[], "Time Start":timestamp, "Peripherals":T12}
  T11 = typedef "Diffuser.ctl" = enum16{"Out of Beam", "In Beam"}
  T12 = typedef "peripherals.ctl" = cluster{"ILX controler":bool, "Zone temperatures":bool, "Andor":bool, "Andor 2":bool, "PI Stage":bool, "AISAS mechanisms":bool, "AISAS Mech.lvclass":refnum<class "AISAS Mech.lvclass">, "Zone temp ref":variant}
  T13 = typedef "Andor Neo Info.ctl" = cluster{"Handle":i32, "Pixel Encoding":string, "AOI Width":i32, "AOI Height":i32, "AOI Stride":i32, "Row Readout Time":dbl, "Frame Readout Time":dbl, "Interframe Time":dbl, "Semaphore":T14, "SerialNumber":string, "Camera Model":string, "Controller ID":string, "Firmware Version":string, "Shutter":string, "BDiv":u8, "Time at Synch":timestamp, "Idx":i32, "PreAmp":string, "Binning":T7, "PixelReadoutRate":string, "Exposure (s)":dbl, "Image Bytes":i64, "Image Pixels":i64, "SpuriousNoiseFilter":bool, "Overlap":bool, "CycleMode":string}
  T14 = typedef "Semaphore RefNum" = refnum<k1>
  T15 = typedef "Cookbook.ctl" = cluster{"Data Type":T16, "Arg 1":sgl, "Arg 2":sgl, "Arg 3":path, "Comments":string}[]
  T16 = typedef "Cbk Data type.ctl" = enum32{"ACQUIRE DATA", "SET DIFFUSER", "CAL-FW", "WAVELENGTH-FW", "INSTR. ROTATION", "SET FOCUS", "DATATYPE", "SET EXPOSURE", "CBK COMMENTS", "MOVE-PI", "MOVE-PI2", "MOVE-PI3", "DWELL TIME"}
  T17 = enum8{"Enabled", "Disabled", "Disabled and Grayed Out"}
  T18 = typedef "Main Program States.ctl" = enum16{"Initialize", "Wait for Event", "Periodic Check", "Update UI", "Update Camera UI", "Load Cookbook", "Run Cookbook", "Snap Images", "Live Preview (Andor)", "Set Filter Wheel", "Set Calibration Wheel", "AISAS Motors on/off", "AISAS Move", "Move AISAS Mechanisms", "Stop", "Change Camera Exposure", "Change Camera Stage Position", "Set Camera AOI", "Andor Adv Settings"}
  T19 = enum16{"Emission Line Filters", "Calibration Polarizers"}
  T20 = typedef "Main Program States.ctl" = enum16{"Initialize", "Wait for Event", "Update UI", "Load Cookbook", "Run Cookbook", "Snap Images", "Live Preview (Andor)", "Set Filter Wheels", "AISAS Motors on/off", "AISAS Move", "Move AISAS Mechanisms", "Stop", "Change Camera Exposure", "Change Camera Stage Position", "Set Camera AOI", "Andor Adv Settings", "Camera Check "}
  T21 = enum16{"1-557.6nm", "2-587.6nm", "3-589.6nm", "4-630.2nm", "5-656.4nm", "6-849.8nm", "7-854.2nm", "8-866.2nm", "9-1083.0nm"}
  T22 = typedef "DialogType.ctl" = u16
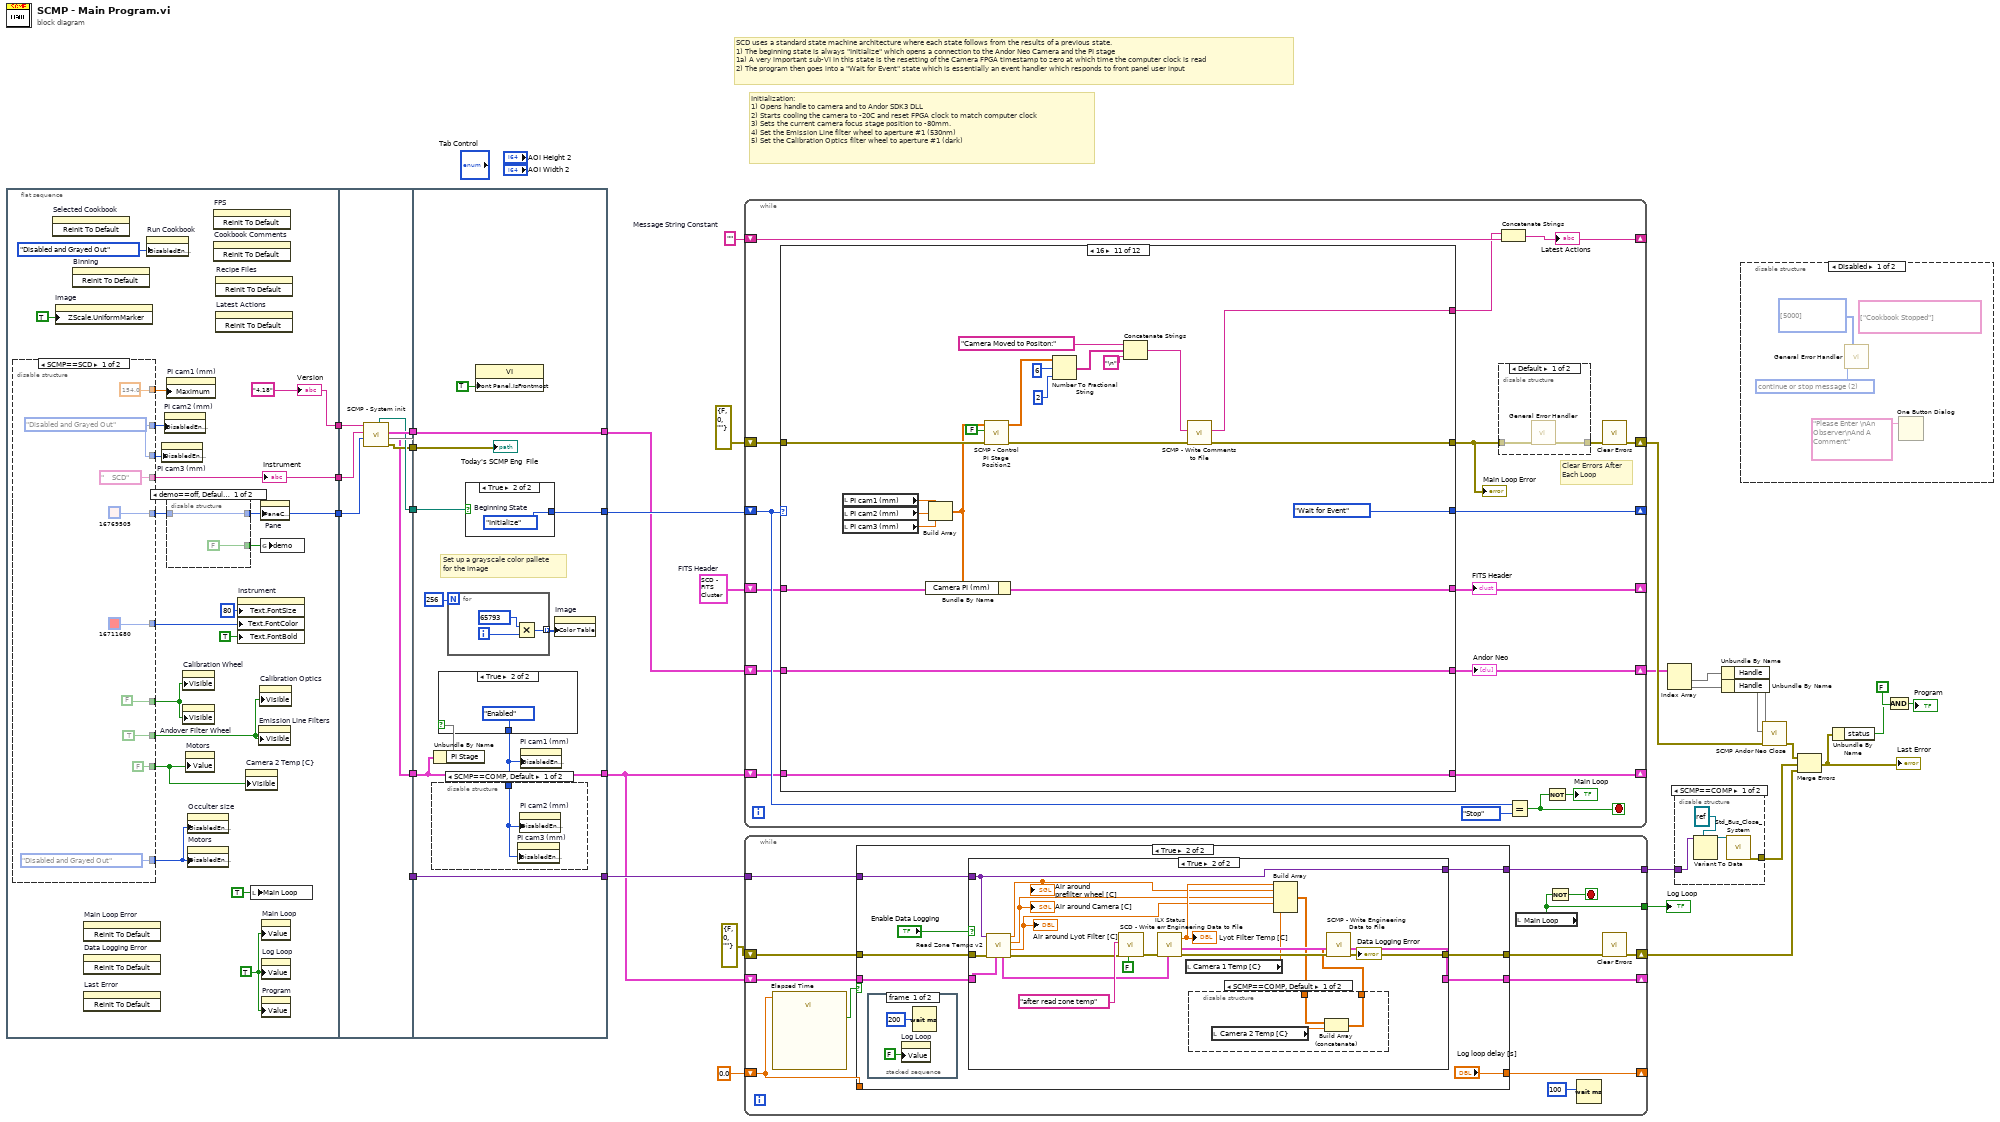
[diagram p0: block diagram]
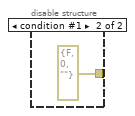
[diagram p2: hidden frame]
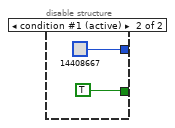
[diagram p3: hidden frame]
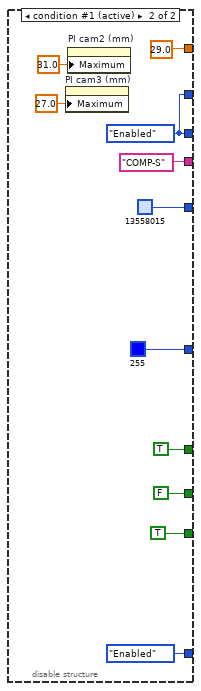
[diagram p4: hidden frame]
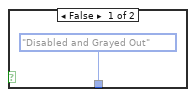
[diagram p6: hidden frame]
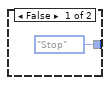
[diagram p7: hidden frame]
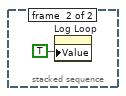
[diagram p10: hidden frame]
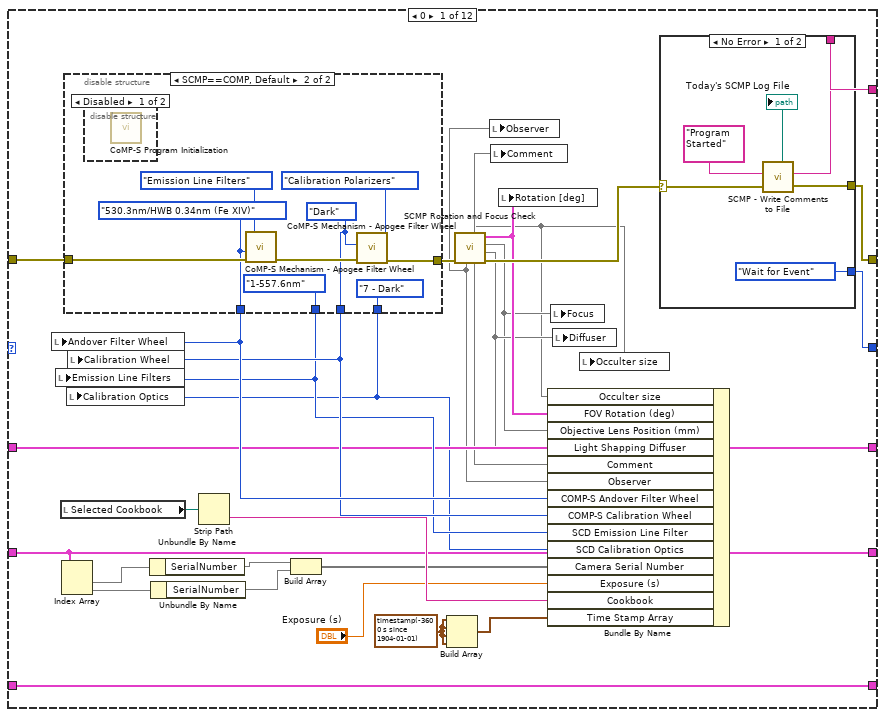
[diagram p13: hidden frame]
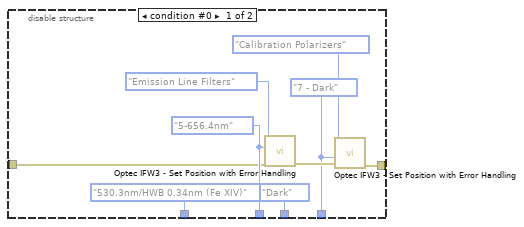
[diagram p14: hidden frame]
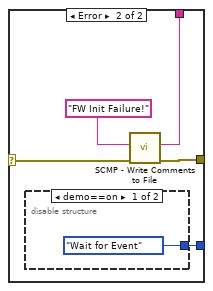
[diagram p16: hidden frame]
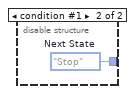
[diagram p17: hidden frame]
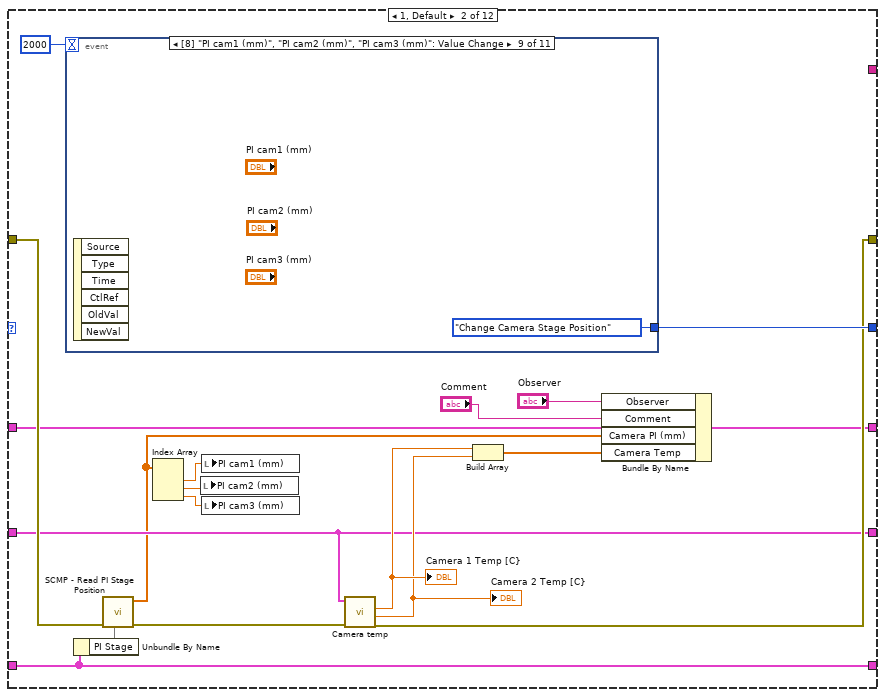
[diagram p18: hidden frame]
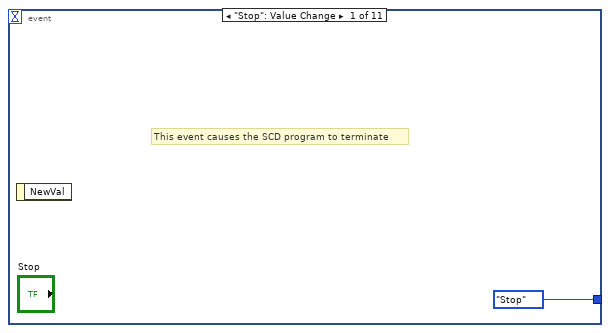
[diagram p19: hidden frame]
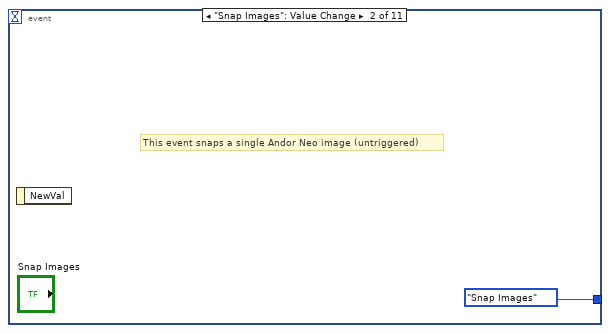
[diagram p20: hidden frame]
diagram:
  w31 = T10 {"Wavelength (nm)"=0.0, "Exposure (s)"=0.0, "Tuning Delay (ms)"=0.0, "Beam Type (-1/1)"=0.0, "Tuning Voltages"=[], "Observer"="", "Light Shapping Diffuser"=enum."Out of Beam", "Comment"="", "Data Type"=0, "Mod Cycles"=0, "SCD Calibration Optics"=enum."1 - Polarizer @0, I+Q", "SCD Emission Line Filter"=enum."1-557.6nm", "Cookbook"="", "COMP-S Calibration Wheel"=enum."Dark", "COMP-S Andover Filter Wheel"=enum."530.3nm/HWB 0.34nm (Fe XIV)", "FOV Rotation (deg)"=0.0, "Objective Lens Position (mm)"=0.0, "Occulter size"=0.0, "Time End"=timestamp(0 s since 1904-01-01), "Acc Exposure (s)"=0.0, "Time Stamp Array"=[], "Camera Serial Number"=[], "Camera Temp"=[], "Camera PI (mm)"=[], "Time Start"=timestamp(3382374145.421875 s since 1904-01-01), "Peripherals"={"ILX controler"=FALSE, "Zone temperatures"=FALSE, "Andor"=FALSE, "Andor 2"=FALSE, "PI Stage"=FALSE, "AISAS mechanisms"=FALSE, "AISAS Mech.lvclass"=refnum, "Zone temp ref"=variant}}  # FITS Header
  w32 = ""  # Message String Constant
  # "Initialization:\n1) Opens handle to camera and to Andor SDK3 DLL\n2) Starts cooling the camera to -20C and reset FPGA clock to match computer clock\n3) Sets the current camera focus stage position to -80mm.\n4) Set the Emission Line filter wheel to aperture #1 (530nm)\n5) Set the Calibration Optics filter wheel to aperture #1 (dark)"
  # "SCD uses a standard state machine architecture where each state follows from the results of a previous state.\n1) The beginning state is always \"Initialize\" which opens a connection to the Andor Neo Camera and the PI stage\n1a) A very important sub-VI in this state is the resetting of the Camera FPGA timestamp to zero at which time the computer clock is read\n2) The program then goes into a \"Wait for Event\" state which is essentially an event handler which responds to front panel user input"
  n1 = flat-sequence {
    tunnel: [w45] -> w23
    tunnel: [w44] -> w22
    tunnel: [w41] -> w20
    tunnel: w23 -> [w82]
    tunnel: w22 -> [w83]
    tunnel: w20 -> [w80]
    tunnel: [w81] -> w17
    tunnel: [w79] -> w16
    tunnel: [w78] -> w15
    tunnel: [w77] -> w9
    tunnel: [w76] -> w7
    tunnel: [w93] -> w6
    tunnel: [w94] -> w21
    tunnel: w17 -> [w94]
    tunnel: w16 -> [w93]
    tunnel: w15 -> [w91]
    tunnel: [w90] -> w14
    tunnel: w9 -> [w89]
    tunnel: [w88] -> w8
    tunnel: w7 -> [w88]
    frame #0 {
      w44 = "4.18" ("Version")
      w47 = TRUE ("Main Loop")
      n2 = disable-structure "Conditional Disable Structure" shown="SCMP==SCD" {
        disable-tunnel: [FALSE ("Visible") TRUE ("Visible")] -> w51
        disable-tunnel: [TRUE ("Visible") FALSE ("Visible")] -> w43
        disable-tunnel: ["    SCD" ("String") "COMP-S" ("String")] -> w45
        disable-tunnel: [u32 16711680 u32 255] -> w48
        disable-tunnel: [u32 16769505 u32 13558015] -> w42
        disable-tunnel: [T17."Disabled and Grayed Out" ("Disabled") T17."Enabled" ("Disabled")] -> w40
        disable-tunnel: [FALSE ("Visible") TRUE ("Visible")] -> w36
        disable-tunnel: [154.0 ("Data Entry Limits:Maximum") 29.0 ("Data Entry Limits:Maximum")] -> w35
        disable-tunnel: [w56 w67] -> w34
        disable-tunnel: [w56 w67] -> w33
        frame condition #0 {
          w56 = T17."Disabled and Grayed Out" ("Disabled")
        }
        frame condition #1 (active) {
          w67 = T17."Enabled" ("Disabled")
          n3 = property on="PI cam3 (mm)" class="DigNum (strict)"("Maximum"=27.0 ("Data Entry Limits:Maximum")) -> ()  [unwired: 2 in, 2 out]
          n4 = property on="PI cam2 (mm)" class="DigNum (strict)"("Maximum"=31.0 ("Data Entry Limits:Maximum")) -> ()  [unwired: 2 in, 2 out]
        }
      }
      "Instrument" <- w45
      n5 = invoke on="Selected Cookbook" class="Path" method="Reinit To Default"() -> ()  [unwired: 3 in, 3 out]
      n6 = property on="Image" class="IntGraph (strict)"("ZScale.UniformMarker"=TRUE ("Z Scale.Uniform Marker Spacing?")) -> ()  [unwired: 2 in, 2 out]
      n7 = invoke on="Binning" class="Enum (strict)" method="Reinit To Default"() -> ()  [unwired: 3 in, 3 out]
      n8 = invoke on="Main Loop Error" class="Clust (strict)" method="Reinit To Default"() -> ()  [unwired: 3 in, 3 out]
      n9 = invoke on="Data Logging Error" class="Clust (strict)" method="Reinit To Default"() -> ()  [unwired: 3 in, 3 out]
      n10 = invoke on="Last Error" class="Clust (strict)" method="Reinit To Default"() -> ()  [unwired: 3 in, 3 out]
      n11 = property on="Run Cookbook" class="Bool"("DisabledEnum"=T17."Disabled and Grayed Out" ("Disabled")) -> ()  [unwired: 2 in, 2 out]
      n12 = property on="PI cam3 (mm)" class="DigNum (strict)"("DisabledEnum"=w33) -> ()  [unwired: 2 in, 2 out]
      n13 = property on="PI cam2 (mm)" class="DigNum (strict)"("DisabledEnum"=w34) -> ()  [unwired: 2 in, 2 out]
      n14 = property on="PI cam1 (mm)" class="DigNum (strict)"("Maximum"=w35) -> ()  [unwired: 2 in, 2 out]
      n15 = disable-structure shown="demo==off, Default" {
        disable-tunnel: [w53 u32 14408667] -> w41
        disable-tunnel: w42 -> [w53 _]
        disable-tunnel: [FALSE ("demo") TRUE ("demo")] -> w39
        frame condition #0 {
        }
        frame condition #1 (active) {
        }
      }
      n16 = property on="Calibration Wheel" class="Enum (strict)"("Visible"=w51) -> ()  [unwired: 2 in, 2 out]
      n17 = property on="Andover Filter Wheel" class="Enum (strict)"("Visible"=w51) -> ()  [unwired: 2 in, 2 out]
      n18 = property on="Motors" class="Bool (strict)"("Value"=w36) -> ()  [unwired: 2 in, 2 out]
      n19 = property on="Occulter size" class="DigNum (strict)"("DisabledEnum"=w40) -> ()  [unwired: 2 in, 2 out]
      n20 = property on="Motors" class="Bool (strict)"("DisabledEnum"=w40) -> ()  [unwired: 2 in, 2 out]
      n21 = invoke on="FPS" class="DigNum (strict)" method="Reinit To Default"() -> ()  [unwired: 3 in, 3 out]
      n22 = invoke on="Cookbook Comments" class="Str" method="Reinit To Default"() -> ()  [unwired: 3 in, 3 out]
      n23 = invoke on="Recipe Files" class="Arr (strict)" method="Reinit To Default"() -> ()  [unwired: 3 in, 3 out]
      n24 = invoke on="Latest Actions" class="Str" method="Reinit To Default"() -> ()  [unwired: 3 in, 3 out]
      n25 = property on="Instrument" class="Str"("Text.FontSize"=u32 80 ("Text.Font:Color"), "Text.FontColor"=w48, "Text.FontBold"=TRUE ("Text.Font:Bold")) -> ()  [unwired: 2 in, 2 out]
      n26 = property on="Camera 2 Temp [C}" class="WFChart (strict)"("Visible"=w36) -> ()  [unwired: 2 in, 2 out]
      n27 = local write "Main Loop"(TRUE ("stop/run")) -> ()
      n28 = property on="Emission Line Filters" class="Enum (strict)"("Visible"=w43) -> ()  [unwired: 2 in, 2 out]
      n29 = property on="Calibration Optics" class="Enum (strict)"("Visible"=w43) -> ()  [unwired: 2 in, 2 out]
      n30 = property on="Pane" class="Pane"("PaneColor"=w41) -> ()  [unwired: 2 in, 2 out]
      n31 = global write "Global demo.vi" "demo"(w39) -> ()
      n32 = property on="Main Loop" class="Bool (strict)"("Value"=w47) -> ()  [unwired: 2 in, 2 out]
      n33 = property on="Log Loop" class="Bool (strict)"("Value"=w47) -> ()  [unwired: 2 in, 2 out]
      n34 = property on="Program" class="Bool (strict)"("Value"=w47) -> ()  [unwired: 2 in, 2 out]
      "Version" <- w44
    }
    frame #1 {
      n35 = call "SCMP - System init.vi"("Pane Color"=w80, "instrument"=w82, 11:w83) -> ("error main"=w77:errorcluster, "Andor array"=w76:T13[], "Peripherals"=w79:T12, 4:w81, "Today's SCMP Engineering File"=w78:path)  [unwired: 2 in, 2 out]
    }
    frame #2 {
      # "Set up a grayscale color pallete for the image"
      n36 = Unbundle By Name(w88) -> ("PI Stage"=w87)
      n37 = case shown="True" w87 {
        tunnel: [T17."Disabled and Grayed Out" ("Disabled") T17."Enabled" ("Disabled")] -> w84
        frame False {
        }
        frame True {
        }
      }
      n38 = disable-structure shown="SCMP==COMP, Default" {
        disable-tunnel: w84 -> [w95 _]
        frame condition #0 (active) {
          n39 = property on="PI cam3 (mm)" class="DigNum (strict)"("DisabledEnum"=w95) -> ()  [unwired: 2 in, 2 out]
          n40 = property on="PI cam2 (mm)" class="DigNum (strict)"("DisabledEnum"=w95) -> ()  [unwired: 2 in, 2 out]
        }
        frame condition #1 {
        }
      }
      n41 = for {
        N: 256 -> [_]
        tunnel: [w97] -> w86 mode=indexing
        i -> [w98]
        n42 = Multiply(x=65793, y=w98) -> (x*y=w97:i32)
      }
      n43 = case shown="True" w91 {
        tunnel: [Main_Program_States."Stop" ("Beginning State") w102] -> w90
        frame False {
        }
        frame True {
          w102 = Main_Program_States."Initialize"  # Beginning State
        }
      }
      n44 = property class="VI"("Front Panel.IsFrontmost"=TRUE ("Front Panel Window:Is Frontmost")) -> ()  [unwired: 2 in, 2 out]
      n45 = property on="PI cam1 (mm)" class="DigNum (strict)"("DisabledEnum"=w84) -> ()  [unwired: 2 in, 2 out]
      n46 = property on="Image" class="IntGraph (strict)"("Color Table"=w86) -> ()  [unwired: 2 in, 2 out]
      "Today's SCMP Eng  File" <- w89
    }
  }
  n47 = while {
    shift-right: [w109] -> _
    shift-left: w14 -> [w119]
    shift-right: [w112] -> w27
    shift-left: errorcluster {"status"=FALSE, "code"=0, "source"=""} ("error out") -> [w118]
    shift-right: [w113] -> _
    shift-left: w32 -> [w115]
    shift-right: [w103] -> _
    shift-left: w31 -> [w117]
    shift-right: [w104] -> w3
    shift-left: w6 -> [w116]
    shift-right: [w105] -> _
    shift-left: w8 -> [w106]
    stop <- w110 stop-if-true
    # "Clear Errors After\nEach Loop"
    n48 = case shown="16" w119 {
      tunnel: [w133 w200 Main_Program_States."Wait for Event" ("Next State") Main_Program_States."Wait for Event" ("Next State") Main_Program_States."Wait for Event" ("Next State") Main_Program_States."Wait for Event" ("Next State") Main_Program_States."Wait for Event" ("Next State") Main_Program_States."Wait for Event" ("Next State") Main_Program_States."Stop" ("Next State") Main_Program_States."Wait for Event" ("Next State") Main_Program_States."Wait for Event" ("Next State") Main_Program_States."Wait for Event" ("Next State")] -> w109
      tunnel: w118 -> [w147 w198 w216 w259 w309 w323 w338 w377 w415 w428 w456 w468]
      tunnel: [w150 w196 w214 w283 w301 w326 w336 w379 w416 w427 w451 w463] -> w107
      tunnel: [w146 _ w231 w285 w310 w325 w340 w381 w419 w429 w457 w465] -> w114
      tunnel: w117 -> [w142 w195 w230 w268 w304 w320 w331 w369 w417 w435 w453 w470]
      tunnel: [w130 w183 w228 w267 w295 w319 w330 w378 w417 w434 w452 w470] -> w103
      tunnel: w116 -> [w126 w187 w229 w269 w296 w318 w339 w380 w418 w422 w454 w459]
      tunnel: [w126 w187 w229 w269 w296 w318 w339 w380 w418 w422 w454 w458] -> w104
      tunnel: [w129 w192 w218 w270 w298 w321 w329 w367 w414 w423 w450 w460] -> w105
      tunnel: w106 -> [w129 w192 w218 w270 w298 w321 w329 w367 w414 w423 w450 w460]
      frame 0 {
        w127 = timestamp(-3600 s since 1904-01-01) ("element")
        n49 = local read "Selected Cookbook"() -> (w149:path)
        n50 = Index Array(array=w126) -> (element #1=w125, element #2=w122)  [unwired: 2 in]
        n51 = disable-structure shown="SCMP==COMP, Default" {
          disable-tunnel: [w159 w166] -> w141
          disable-tunnel: w147 -> [w151 w167]
          disable-tunnel: [w153 SCD_-_EDT_-_Emission_Line_Filter_Wheel."1-557.6nm" ("Emission Line Filters")] -> w143
          disable-tunnel: [Emission_Line_Filter_Wheel."530.3nm/HWB 0.34nm (Fe XIV)" ("Emission Line Filters [530.3 nm]") w162] -> w145
          disable-tunnel: [Polarization_Optics_Filter_Wheel."Dark" ("Calibration Polarizer \nFilter Wheel [Dark]") w161] -> w144
          disable-tunnel: [w152 SCD_-_Calibration_Optics_Filter_Wheel."7 - Dark" ("Calibration Optics")] -> w132
          frame condition #0 {
            w152 = SCD_-_Calibration_Optics_Filter_Wheel."7 - Dark" ("SCD Calibration Optics")
            w153 = T21."5-656.4nm" ("Emission Line Filter")
            n52 = call "Optec IFW3 - Set Position with Error Handling.vi"("error in"=w151, "Emission Line Filter"=w153, "Filter Wheel Selector"=T19."Emission Line Filters") -> ("error out"=w158:errorcluster)  [unwired: 6 in, 2 out]
            n53 = call "Optec IFW3 - Set Position with Error Handling.vi"("error in"=w158, "SCD Calibration Optics"=w152, "Filter Wheel Selector"=T19."Calibration Polarizers") -> ("error out"=w159:errorcluster)  [unwired: 6 in, 2 out]
          }
          frame condition #1 (active) {
            w161 = Polarization_Optics_Filter_Wheel."Dark" ("Calibration Polarizer \nFilter Wheel [Dark]")
            w162 = Emission_Line_Filter_Wheel."530.3nm/HWB 0.34nm (Fe XIV)" ("Emission Line Filters [530.3 nm]")
            n54 = disable-structure shown="Disabled" {
              frame Disabled {
                n55 = call "CoMP-S Program Initialization.vi"() -> ()  [unwired: 8 in, 4 out]
              }
              frame Enabled {
              }
            }
            n56 = call "CoMP-S Mechanism - Apogee Filter Wheel.vi"("error in (no error)"=w167, "Emission Line Filters [530.3 nm]"=w162, "Filter Wheel Selector"=T19."Emission Line Filters") -> ("error out"=w165:errorcluster)  [unwired: 5 in, 3 out]
            n57 = call "CoMP-S Mechanism - Apogee Filter Wheel.vi"("error in (no error)"=w165, "Calibration Polarizer Filters [Dark]"=w161, "Filter Wheel Selector"=T19."Calibration Polarizers") -> ("error out"=w166:errorcluster)  [unwired: 5 in, 3 out]
          }
        }
        n58 = local write "Andover Filter Wheel"(w145) -> ()
        n59 = local write "Emission Line Filters"(w143) -> ()
        n60 = local write "Calibration Optics"(w132) -> ()
        n61 = local write "Calibration Wheel"(w144) -> ()
        n62 = Unbundle By Name(w125) -> ("SerialNumber"=w124)
        n63 = Unbundle By Name(w122) -> ("SerialNumber"=w121)
        n64 = Strip Path(path=w149) -> (name=w148:string)  [unwired: 1 out]
        n65 = Build Array(w124, w121) -> (w123:void[])
        n66 = Build Array(w127, w127, w127, w127) -> (w128:timestamp[])
        n67 = call "SCMP Rotation and Focus Check.vi"("error in"=w141) -> ("error out"=w140:errorcluster, 1:w138, 2:w135, "FITS Header Out"=w139:T10, 4:w136, 5:w134, 6:w137)  [unwired: 4 in]
        n68 = local write "Observer"(w137) -> ()
        n69 = local write "Comment"(w136) -> ()
        n70 = local write "Rotation [deg]"(w139) -> ()
        n71 = Bundle By Name(cluster=w142, "Occulter size"=w134, "FOV Rotation (deg)"=w139, "Objective Lens Position (mm)"=w135, "Light Shapping Diffuser"=w138, "Comment"=w136, "Observer"=w137, "COMP-S Andover Filter Wheel"=w145, "COMP-S Calibration Wheel"=w144, "SCD Emission Line Filter"=w143, "SCD Calibration Optics"=w132, "Camera Serial Number"=w123, "Exposure (s)"="Exposure (s)", "Cookbook"=w148, "Time Stamp Array"=w128) -> (w130:T10)
        n72 = local write "Focus"(w135) -> ()
        n73 = local write "Diffuser"(w138) -> ()
        n74 = local write "Occulter size"(w134) -> ()
        n75 = case shown="No Error" w140 {
          selector: w140 -> [w171 w177]
          tunnel: [w174 w179] -> w146
          tunnel: [Main_Program_States."Wait for Event" ("Next State") w178] -> w133
          tunnel: [w170 w176] -> w150
          frame No Error {
            n76 = call "SCMP - Write Comments to File.vi"("error in"=w171, "data"="Program Started") -> ("error out"=w170:errorcluster, "Last Log Entry"=w174:string, "Today's SCMP Log File"=→"Today's SCMP Log File":path)  [unwired: 6 in, 1 out]
          }
          frame Error {
            n77 = disable-structure shown="demo==on" {
              disable-tunnel: [Main_Program_States."Wait for Event" ("Next State") w181] -> w178
              frame condition #0 (active) {
              }
              frame condition #1 {
                w181 = Main_Program_States."Stop"  # Next State
              }
            }
            n78 = call "SCMP - Write Comments to File.vi"("error in"=w177, "data"="FW Init Failure!") -> ("error out"=w176:errorcluster, "Last Log Entry"=w179:string)  [unwired: 6 in, 2 out]
          }
        }
      }
      frame 1, Default {
        n79 = event shown="[8] \"PI cam1 (mm)\", \"PI cam2 (mm)\", \"PI cam3 (mm)\": Value Change" {
          selector: _ -> [_ _ _ _ _ _ _ _ _ _ _]
          dyn-events: _ -> [_ _ _ _ _ _ _ _ _ _ _]
          timeout: 2000 -> [_ _ _ _ _ _ _ _ _ _ _]
          tunnel: [Main_Program_States."Stop" ("Next State") Main_Program_States."Snap Images" ("Next State") Main_Program_States."Wait for Event" ("Next State") Main_Program_States."Live Preview (Andor)" ("Next State") Main_Program_States."Load Cookbook" ("Next State") Main_Program_States."Run Cookbook" ("Next State") Main_Program_States."Set Filter Wheels" ("Next State") Main_Program_States."Move AISAS Mechanisms" ("Next State") Main_Program_States."Change Camera Stage Position" ("Next State") Main_Program_States."Set Camera AOI" ("Next State") Main_Program_States."Change Camera Exposure" ("Next State")] -> w200
          event "Stop": Value Change {
            # "This event causes the SCD program to terminate"
            n80 = event-data() -> ()  [unwired: 1 in, 1 out]
          }
          event "Snap Images": Value Change {
            # "This event snaps a single Andor Neo image (untriggered)"
            n81 = event-data() -> ()  [unwired: 1 in, 1 out]
          }
          event Timeout {
            # "I commented out this 'file read' operation as it tends to slow things\ndown when it gets large.  The \"Latest Actions\" indicator has the same\ninformation and requires less CPU power."
            n82 = event-data() -> ()  [unwired: 1 in, 3 out]
            n83 = disable-structure shown="Disabled" {
              frame Disabled {
                n84 = local read "Today's SCMP Log File"() -> (w205:path)
                n85 = Read from Text File(file (use dialog)=w205) -> (text=→"Continually Read Log File":string)  [unwired: 3 in, 3 out]
              }
              frame Enabled {
              }
            }
          }
          event "Live Preview (Andor)": Value Change {
            # "This event streams images from the Andor Neo camera\nto the front panel user interface (untriggered)"
            n86 = event-data() -> ()  [unwired: 1 in, 4 out]
          }
          event "Load Cookbook": Value Change {
            # "This event lets an observer select a cookbook to 'run'"
            n87 = event-data() -> ()  [unwired: 1 in, 1 out]
          }
          event "Run Cookbook": Value Change {
            # "This event runs a previously loaded cookbook sequence\nCookbooks can take many minutes to run..."
            n88 = event-data() -> ()  [unwired: 1 in, 1 out]
          }
          event "Set Filter Wheels": Value Change {
            # "This event allows an operator to manually set the position of\nboth SCD filter wheels.  \n1) Andover Pre-Filter"
            n89 = event-data() -> ()  [unwired: 1 in, 6 out]
          }
          event "Move AISAS Mechanisms": Value Change {
            n90 = event-data() -> ()  [unwired: 1 in, 6 out]
          }
          event Value Change {
            n91 = event-data() -> ()  [unwired: 1 in, 6 out]
          }
          event Value Change {
            n92 = event-data() -> ()  [unwired: 1 in, 6 out]
          }
          event "Exposure (s)": Value Change {
            n93 = event-data() -> ()  [unwired: 1 in, 6 out]
          }
        }
        n94 = Unbundle By Name(w192) -> ("PI Stage"=w191)
        n95 = call "SCMP - Read PI Stage Position.vi"("Enable"=w191, "error in (no error)"=w198) -> ("error out"=w197:errorcluster, "Output Array"=w182:dbl[])  [unwired: 8 in]
        n96 = Index Array(array=w182) -> (element #1=w185:dbl, element #2=w186:dbl, element #3=w184:dbl)  [unwired: 3 in]
        n97 = local write "PI cam2 (mm)"(w186) -> ()
        n98 = local write "PI cam1 (mm)"(w185) -> ()
        n99 = local write "PI cam3 (mm)"(w184) -> ()
        n100 = call "Camera temp.vi"("error in (no error)"=w197, "Andor Neo"=w187) -> ("error out"=w196:errorcluster, "Camera 2 Temp [C}"=w189:dbl, "Camera 1 Temp [C}"=w190:dbl)  [unwired: 7 in]
        "Camera 1 Temp [C}" <- w190
        "Camera 2 Temp [C}" <- w189
        n101 = Build Array(w190, w189) -> (w188:dbl[])
        n102 = Bundle By Name(cluster=w195, "Observer"="Observer", "Comment"="Comment", "Camera PI (mm)"=w182, "Camera Temp"=w188) -> (w183:T10)
      }
      frame 5 {
        n103 = call "SCMP - Read Cookbook.vi"("error in"=w216) -> ("error out"=w225:errorcluster, "Recipe Files"=→"Recipe Files":string[], "# of Recipes"=w222:i16, "Cookbook"=→"Cookbook":T15, "min Cookbook Exposure [s]"=w221:dbl, "Selected Cookbook"=w217:path, "Cookbook Comments"=→"Cookbook Comments":string)  [unwired: 4 in]
        "max Cookbook Exposure [s]" <- w221
        "Selected Cookbook" <- w217
        n104 = case shown="No Error" w225 {
          selector: w225 -> [w238 w244]
          tunnel: w222 -> [w241 _]
          tunnel: w217 -> [w239 w247]
          tunnel: [w240 w245] -> w232
          tunnel: [w238 w244] -> w226
          frame No Error {
            n105 = Strip Path(path=w239) -> (name=w236:string)  [unwired: 1 out]
            "cbk name" <- w236
            n106 = property on="Run Cookbook" class="Bool"("DisabledEnum"=T17."Enabled" ("Disabled")) -> ()  [unwired: 2 in, 2 out]
            n107 = Concatenate Strings("Loaded Cookbook" ("data"), "\t", w236) -> (w240:string)
            "# of Recipes" <- w241
          }
          frame Error {
            n108 = Strip Path(path=w247) -> (name=w246:string)  [unwired: 1 out]
            n109 = Concatenate Strings("Error Loading Cookbook" ("data"), "\t", w246) -> (w245:string)
            n110 = property on="Run Cookbook" class="Bool"("DisabledEnum"=T17."Disabled and Grayed Out" ("Disabled")) -> ()  [unwired: 2 in, 2 out]
          }
        }
        n111 = call "SCMP - Set Exp and Check FPS.vi"("Exposure [s]"=w221) -> ("FPS"=w219:dbl)  [unwired: 9 in, 1 out]
        n112 = local write "FPS"(w219) -> ()
        n113 = Strip Path(path=w217) -> (name=w227:string)  [unwired: 1 out]
        n114 = call "SCMP - Write Comments to File.vi"("error in"=w226, "data"=w232) -> ("error out"=w215:errorcluster, "Last Log Entry"=w231:string)  [unwired: 6 in, 2 out]
        n115 = Bundle By Name(cluster=w230, "Cookbook"=w227) -> (w228:T10)
        n116 = call <vilib>:"Clear Errors.vi"("error in (no error)"=w215) -> ("error out"=w214:errorcluster)  [unwired: 5 in, 1 out]
      }
      frame 6 {
        n117 = flat-sequence {
          tunnel: [w294] -> w258
          tunnel: w259 -> [w294]
          tunnel: [w293] -> w254
          frame #0 {
            n118 = Get Date/Time In Seconds() -> (seconds since 1Jan1904=w293:timestamp)
          }
        }
        n119 = local read "Motors"() -> (w266:bool)
        n120 = local read "Cookbook"() -> (w273:T15)
        n121 = Unbundle By Name(w270) -> ("PI Stage"=w265)
        n122 = call "SCMP - Run Cookbook.vi"("Cookbook"=w273, "Mod/Seq"="Mod/Seq", "Save to FITS?"="Save Data to FITS?", "limit max FPS to:"="FPS", "Motors"=w266, 9:w265, "Error in"=w258, "Andor Neo"=w269, "FITS Header In"=w268) -> ("Result"=w252:string, "FITS Path Out"=→"FITS Path from Last Recipe Acquiring Data":path, "Updated Header"=w267:T10, "Error out"=w257:errorcluster)  [unwired: 3 in]
        n123 = Unbundle By Name(w267) -> ("COMP-S Calibration Wheel"=w280:T6, "COMP-S Andover Filter Wheel"=w279:T5, "SCD Calibration Optics"=w278:T3, "SCD Emission Line Filter"=w277:T9, "Exposure (s)"=w276:dbl, "Light Shapping Diffuser"=w275:T11, "FOV Rotation (deg)"=w274:dbl, "Objective Lens Position (mm)"=w272:T4, "Camera PI (mm)"=w264:dbl[])
        n124 = flat-sequence {
          tunnel: [w292] -> w256
          tunnel: w257 -> [w292]
          tunnel: [w291] -> w255
          frame #0 {
            n125 = Get Date/Time In Seconds() -> (seconds since 1Jan1904=w291:timestamp)
          }
        }
        n126 = Subtract(x=w255, y=w254) -> (x-y=w253:dbl)
        n127 = Index Array(array=w264) -> (element #1=w263:dbl, element #2=w262:dbl, element #3=w261:dbl)  [unwired: 3 in]
        n128 = Format Date/Time String(time format string (%c)="%M:%S] ", seconds (now)=w253) -> (date/time string=w250:string)  [unwired: 1 in]
        n129 = local write "Calibration Wheel"(w280) -> ()
        n130 = local write "Andover Filter Wheel"(w279) -> ()
        n131 = local write "Calibration Optics"(w278) -> ()
        n132 = local write "Emission Line Filters"(w277) -> ()
        n133 = local write "Exposure (s)"(w276) -> ()
        n134 = local write "Rotation [deg]"(w274) -> ()
        n135 = local write "PI cam2 (mm)"(w262) -> ()
        n136 = local write "PI cam3 (mm)"(w261) -> ()
        n137 = local write "PI cam1 (mm)"(w263) -> ()
        n138 = local write "Focus"(w272) -> ()
        n139 = local write "Diffuser"(w275) -> ()
        n140 = local read "cbk name"() -> (w286:string)
        n141 = Concatenate Strings("Run Cookbook" ("data"), "\t", w286, "\r", w252, " [" ("string"), w250) -> (w288:string)
        n142 = call "SCMP - Write Comments to File.vi"("error in"=w256, "data"=w288) -> ("error out"=w283:errorcluster, "Last Log Entry"=w285:string)  [unwired: 6 in, 2 out]
      }
      frame 7 {
        n143 = Bundle By Name(cluster=w304, "Wavelength (nm)"=0.0) -> (w295:T10)
        n144 = local read "Save Data to FITS? (F)"() -> (w297:bool)
        n145 = call "Andor Neo - Snap Single Image.vi"("FITS Header"=w295, "error in"=w309, "Andor Neo"=w296, "Save Data to FITS? (F)"=w297) -> ("error out"=w300:errorcluster, "Image Graph 2"=→"Histogram Graph":u16[][], "Image Graph"=→"Mean ADU":u16[][], 3:w303, "Snapshot FITS arr"=→"Snapshot FITS File Path":path[], "FPGA Timestamp arr"=→"Timestamp":timestamp[])  [unwired: 2 in]
        "Image" <- w303
        n146 = call "SCD - Determine Image Sharpness from 2D Derivative.vi"("Image In"=w303) -> ("Sharpness"=→"Image Sharpness":dbl)  [unwired: 9 in, 1 out]
        n147 = call "SCMP - Write Comments to File.vi"("error in"=w300, "data"="Snap Single Image") -> ("error out"=w301:errorcluster, "Last Log Entry"=w310:string)  [unwired: 6 in, 2 out]
      }
      frame 8 {
        n148 = call "SCMP Andor Neo - Live ext trigger.vi"("FITS Header in"=w320, "error in"=w323, "Andor Neo"=w318, "Save Data? (F)"="Save Data to FITS? (F)") -> ("error out"=w324:errorcluster, "FITS Header out"=w319:T10)  [unwired: 6 in]
        n149 = disable-structure shown="Disabled" {
          frame Disabled {
            n150 = call "SCMP Andor Neo - Snap Single Image (Cont).vi"() -> ()  [unwired: 10 in, 2 out]
          }
          frame Enabled {
          }
        }
        n151 = Unbundle By Name(w319) -> ("Exposure (s)"=w317:dbl, "Camera PI (mm)"=w316:dbl[])
        n152 = Index Array(array=w316) -> (element #1=w315:dbl, element #2=w314:dbl, element #3=w313:dbl)  [unwired: 3 in]
        n153 = local write "Exposure (s)"(w317) -> ()
        n154 = local write "PI cam1 (mm)"(w315) -> ()
        n155 = local write "PI cam2 (mm)"(w314) -> ()
        n156 = local write "PI cam3 (mm)"(w313) -> ()
        n157 = call "SCMP - Write Comments to File.vi"("error in"=w324, "data"="Live Preview Images") -> ("error out"=w326:errorcluster, "Last Log Entry"=w325:string)  [unwired: 6 in, 2 out]
      }
      frame 7 {
        w341 = "\t"
        n158 = disable-structure shown="SCMP==COMP, Default" {
          disable-tunnel: w338 -> [w355 w362]
          disable-tunnel: [w353 w361] -> w337
          disable-tunnel: [w352 w363] -> w335
          disable-tunnel: [w351 w360] -> w332
          disable-tunnel: [w349 w359] -> w330
          disable-tunnel: w331 -> [w350 w358]
          frame condition #0 {
            n159 = disable-structure shown="Disabled" {
              frame Disabled {
                # "old filter wheel vi"
                n160 = call "Optec IFW3 - Standalone.vi"() -> ()  [unwired: 11 in, 1 out]
              }
              frame Enabled {
              }
            }
            n161 = Bundle By Name(cluster=w350, "SCD Calibration Optics"="Calibration Optics", "SCD Emission Line Filter"="Emission Line Filters") -> (w349:T10)
            n162 = call "Optec IFW3 - Set Position with Error Handling.vi"("error in"=w355, "Emission Line Filter"="Emission Line Filters", "Filter Wheel Selector"=T19."Emission Line Filters") -> ("error out"=w354:errorcluster, "Actual Position (1-9)"=w353:i32)  [unwired: 6 in, 1 out]
            n163 = call "Optec IFW3 - Set Position with Error Handling.vi"("error in"=w354, "SCD Calibration Optics"="Calibration Optics", "Filter Wheel Selector"=T19."Calibration Polarizers") -> ("error out"=w352:errorcluster, "Actual Position (1-9)"=w351:i32)  [unwired: 6 in, 1 out]
          }
          frame condition #1 (active) {
            n164 = Bundle By Name(cluster=w358, "COMP-S Calibration Wheel"="Calibration Wheel", "COMP-S Andover Filter Wheel"="Andover Filter Wheel") -> (w359:T10)
            n165 = call "CoMP-S Mechanism - Apogee Filter Wheel.vi"("error in (no error)"=w362, "Emission Line Filters [530.3 nm]"="Andover Filter Wheel", "Filter Wheel Selector"=T19."Emission Line Filters") -> ("error out"=w365:errorcluster, "Position"=w361:i32)  [unwired: 5 in, 2 out]
            n166 = call "CoMP-S Mechanism - Apogee Filter Wheel.vi"("error in (no error)"=w365, "Calibration Polarizer Filters [Dark]"="Calibration Wheel", "Filter Wheel Selector"=T19."Calibration Polarizers") -> ("error out"=w363:errorcluster, "Position"=w360:i32)  [unwired: 5 in, 2 out]
          }
        }
        n167 = Number To Decimal String(number=w332) -> (decimal integer string=w342:string)  [unwired: 1 in]
        n168 = Number To Decimal String(number=w337) -> (decimal integer string=w333:string)  [unwired: 1 in]
        n169 = Concatenate Strings("Updated Calibration & Filter wheel position:" ("data"), w341, w342, w341, w333) -> (w334:string)
        n170 = call "SCMP - Write Comments to File.vi"("error in"=w335, "data"=w334) -> ("error out"=w336:errorcluster, "Last Log Entry"=w340:string)  [unwired: 6 in, 2 out]
      }
      frame 13 {
        n171 = call "SCMP - cmp instr val.vi"("FITS Header in"=w369, "Diffuser"="Diffuser", "error in (no error)"=w377, "Occulter size"="Occulter size", "Rotation"="Rotation [deg]", "Focus"="Focus") -> ("error out"=w376:errorcluster, "value changed arr"=w370:bool[], "value changed"=w371:bool)  [unwired: 2 in]
        n172 = case shown="True" w371 {
          tunnel: ["" ("Entire Log File") w404] -> w381
          tunnel: [w385 w410] -> w379
          tunnel: [w384 w407] -> w378
          tunnel: w376 -> [w385 w403]
          tunnel: w369 -> [w384 w405]
          tunnel: "Diffuser" -> [_ w392]
          tunnel: "Focus" -> [_ w399]
          tunnel: "Rotation [deg]" -> [_ w398]
          tunnel: "Occulter size" -> [_ w394]
          tunnel: w370 -> [_ w401]
          tunnel: w369 -> [_ w393]
          tunnel: "Motors" -> [_ w388]
          frame False {
          }
          frame True {
            w408 = "\t"
            n173 = call "SCMP -Move AISAS.vi"("FITS Header in"=w393, "Motors"=w388, "Diffuser in"=w392, "error in (no error)"=w403, "value changed arr"=w401, "Rotation in"=w398, "Focus in"=w399) -> ("error out"=w402:errorcluster, "New Rotation"=w389:dbl, "New Focus"=w390:T4, "New Diffuser"=w391:T11)  [unwired: 1 in]
            n174 = local write "Diffuser"(w391) -> ()
            n175 = local write "Focus"(w390) -> ()
            n176 = local write "Rotation [deg]"(w389) -> ()
            n177 = call "SCMP - update instr val.vi"("FITS Header in"=w405, "Diffuser"=w391, "error in (no error)"=w402, "Occulter size"=w394, "Rotation [deg]"=w389, "Focus"=w390) -> ("error out"=w406:errorcluster, "FITS Header out"=w407:T10)  [unwired: 4 in]
            n178 = call "SCMP write init xml.vi"(7:w391, "error in (no error)"=w406, 9:w394, 10:w389, "FITS Header In"=w390) -> ("error out"=w409:errorcluster)  [unwired: 5 in, 1 out]
            n179 = Number To Decimal String(number=w391) -> (decimal integer string=w411:string)  [unwired: 1 in]
            n180 = Number To Fractional String(number=w390, precision (6)=i16 2) -> (F-format string=w400:string)  [unwired: 2 in]
            n181 = Number To Fractional String(number=w389, precision (6)=i16 1) -> (F-format string=w396:string)  [unwired: 2 in]
            n182 = Number To Fractional String(number=w394, precision (6)=i16 2) -> (F-format string=w395:string)  [unwired: 2 in]
            n183 = Concatenate Strings("Instrument set to (Diff/Foc/Rot/Occ):" ("string"), w408, w411, w408, w400, w408, w396, w408, w395, w408) -> (w412:string)
            n184 = call "SCMP - Write Comments to File.vi"("error in"=w409, "data"=w412) -> ("error out"=w410:errorcluster, "Last Log Entry"=w404:string)  [unwired: 6 in, 2 out]
          }
        }
      }
      frame 14 {
        n185 = call "SCMP - Write Comments to File.vi"("error in"=w415, "data"="Program Terminated") -> ("error out"=w416:errorcluster, "Last Log Entry"=w419:string)  [unwired: 6 in, 2 out]
      }
      frame 15 {
        n186 = local read "Exposure (s)"() -> (w424:dbl)
        n187 = call "Andor Neo - Set Exposure Time.vi"(6:w422, "error in (no error)"=w428, "Desired Exposure (s)"=w424) -> ("error out"=w426:errorcluster, "True Exposure (s)"=w425:dbl)  [unwired: 6 in, 1 out]
        n188 = local write "Exposure (s)"(w425) -> ()
        n189 = Bundle By Name(cluster=w435, "Exposure (s)"=w425) -> (w434:T10)
        n190 = Number To Fractional String(number=w425) -> (F-format string=w432:string)  [unwired: 3 in]
        n191 = Concatenate Strings("Camera Exposure Changed to " ("data"), w432, " seconds" ("string")) -> (w430:string)
        n192 = call "SCMP - Write Comments to File.vi"("error in"=w426, "data"=w430) -> ("error out"=w427:errorcluster, "Last Log Entry"=w429:string)  [unwired: 6 in, 2 out]
      }
      frame 16 {
        n193 = local read "PI cam1 (mm)"() -> (w441:T2)
        n194 = local read "PI cam2 (mm)"() -> (w440:T2)
        n195 = local read "PI cam3 (mm)"() -> (w439:T2)
        n196 = Build Array(w441, w440, w439) -> (w438:T2[])
        n197 = Bundle By Name(cluster=w453, "Camera PI (mm)"=w438) -> (w452:T10)
        n198 = call "SCMP - Control PI Stage Position2.vi"("error in"=w456, "Absolute (F) or \nRelative (T) Move"=FALSE ("Absolute (F) or \nRelative (T) Move"), "set values"=w438) -> ("error out"=w443:errorcluster, "Position"=w442:dbl[])  [unwired: 6 in, 1 out]
        n199 = Number To Fractional String(number=w442, width (-)=i16 6, precision (6)=i16 2) -> (F-format string=w448:string[])  [unwired: 1 in]
        n200 = Concatenate Strings("Camera Moved to Positon:" ("Recent Log"), w448, "\n" ("string")) -> (w447:string)
        n201 = call "SCMP - Write Comments to File.vi"("error in"=w443, "data"=w447) -> ("error out"=w451:errorcluster, "Last Log Entry"=w457:string)  [unwired: 6 in, 2 out]
      }
      frame 17 {
        n202 = call "Andor Neo - Set Binning.vi"("Andor Neo"=w459, "error in"=w468, "Binning"="Binning") -> ("error out"=w462:errorcluster, "Andor Neo out"=w458:T13[])  [unwired: 7 in]
        n203 = property on="Binning" class="Enum (strict)"() -> ("RingText.Text"=w461:string)  [unwired: 2 in, 2 out]
        n204 = Concatenate Strings("Set Camera Binning: " ("Recent Log"), w461) -> (w466:string)
        n205 = call "SCMP - Write Comments to File.vi"("error in"=w462, "data"=w466) -> ("error out"=w463:errorcluster, "Last Log Entry"=w465:string)  [unwired: 6 in, 2 out]
      }
    }
    "FITS Header" <- w103
    "Main Loop Error" <- w107
    "Andor Neo" <- w104
    n206 = disable-structure shown="Default" {
      disable-tunnel: [w472 w473] -> w108
      disable-tunnel: w107 -> [w471 w473]
      frame condition #0 {
        n207 = call <vilib>:"General Error Handler.vi"("error in (no error)"=w471) -> ("error out"=w472:errorcluster)  [unwired: 10 in, 4 out]
      }
      frame condition #1 (active) {
      }
    }
    n208 = Concatenate Strings(w114, w115) -> (w113:string)
    "Latest Actions" <- w113
    n209 = Equal?(x=w119, y=Main_Program_States."Stop" ("States")) -> (x = y?=w110:bool)
    n210 = Not(x=w110) -> (.not. x?=→"Main Loop":bool)
    n211 = call <vilib>:"Clear Errors.vi"("error in (no error)"=w108) -> ("error out"=w112:errorcluster)  [unwired: 5 in, 1 out]
  }
  n212 = while {
    shift-right: [w475] -> w26
    shift-left: errorcluster {"status"=FALSE, "code"=0, "source"=""} ("error out") -> [w485]
    tunnel: w21 -> [w486]
    tunnel: [w484] -> w29
    shift-right: [w481] -> _
    shift-left: 0.0 ("Time Target (s)") -> [w478]
    tunnel: [w479] -> w24
    shift-right: [w477] -> _
    shift-left: w8 -> [w476]
    stop <- w483 stop-if-true
    n213 = call "Elapsed Time"("Time Target (s)"=w478) -> ("Time has Elapsed"=w482:bool)  [unwired: 11 in, 7 out]
    n214 = case shown="True" w482 {
      tunnel: w486 -> [w488 w498]
      tunnel: w485 -> [w489 w496]
      tunnel: [w489 w495] -> w474
      tunnel: w478 -> [w490 _]
      tunnel: [w490 "Log loop delay [s]"] -> w481
      tunnel: [w488 w493] -> w479
      tunnel: w476 -> [w487 w492]
      tunnel: [w487 w491] -> w477
      frame False {
      }
      frame True {
        n215 = stacked-sequence {
          frame #0 {
            n216 = property on="Log Loop" class="Bool (strict)"("Value"=FALSE ("Log Loop")) -> ()  [unwired: 2 in, 2 out]
            n217 = Wait (ms)(milliseconds to wait=u32 200) -> ()  [unwired: 1 out]
          }
          frame #1 {
            n218 = property on="Log Loop" class="Bool (strict)"("Value"=TRUE ("Log Loop")) -> ()  [unwired: 2 in, 2 out]
          }
        }
        n219 = case shown="True" "Enable Data Logging" {
          tunnel: w496 -> [w504 w517]
          tunnel: [w504 w509] -> w495
          tunnel: w498 -> [w503 w518]
          tunnel: [w503 w518] -> w493
          tunnel: w492 -> [w502 w511]
          tunnel: [w502 w512] -> w491
          frame False {
          }
          frame True {
            n220 = call "Read Zone Temps v2.vi"("Peripherals"=w511, "error in"=w517, 11:w518) -> ("error out"=w516:errorcluster, "Air Temp [C]"=w513:dbl, "Camera Body [C]"=w519:sgl, "Pre-Filter Temp [C}"=w514:sgl, "Peripherals out"=w510:T12)  [unwired: 4 in]
            "Air around Camera [C]" <- w519
            "Air around \nprefilter wheel [C]" <- w514
            "Air around Lyot Filter [C]" <- w513
            n221 = call "SCD - Write err Engineering Data to File.vi"("debug"=FALSE, "error in"=w516, "message"="after read zone temp") -> ("error out"=w508:errorcluster)  [unwired: 8 in]
            n222 = call "ILX Status.vi"("Peripherals in"=w510, "error in"=w508) -> ("error out"=w515:errorcluster, "Temperature"=w522:dbl, "Peripherals out"=w512:T12)  [unwired: 4 in, 3 out]
            "Lyot Filter Temp [C]" <- w522
            n223 = local read "Camera 1 Temp [C}"() -> (w507:dbl)
            n224 = Build Array(w522, w514, w519, w513, w507) -> (w506:dbl[])
            n225 = disable-structure shown="SCMP==COMP, Default" {
              disable-tunnel: w506 -> [w524 w526]
              disable-tunnel: [w523 w526] -> w505
              frame condition #0 (active) {
                n226 = local read "Camera 2 Temp [C}"() -> (w525:dbl)
                n227 = Build Array (concatenate)(w524, w525) -> (w523:dbl[])
              }
              frame condition #1 {
              }
            }
            n228 = call "SCMP - Write Engineering Data to File.vi"("error in"=w515, "Temp Data"=w505) -> ("error out"=w509:errorcluster)  [unwired: 6 in, 3 out]
            "Data Logging Error" <- w509
          }
        }
      }
    }
    n229 = local read "Main Loop"() -> (w484:bool)
    n230 = Not(x=w484) -> (.not. x?=w483:bool)
    n231 = Wait (ms)(milliseconds to wait=u32 100) -> ()  [unwired: 1 out]
    n232 = call <vilib>:"Clear Errors.vi"("error in (no error)"=w474) -> ("error out"=w475:errorcluster)  [unwired: 5 in, 1 out]
  }
  "Log Loop" <- w29
  n233 = Index Array(array=w3) -> (element #1=w5, element #2=w4)  [unwired: 2 in]
  n234 = disable-structure shown="SCMP==COMP" {
    disable-tunnel: [w530 errorcluster {"status"=FALSE, "code"=0, "source"=""} ("error out")] -> w25
    disable-tunnel: w24 -> [w529 _]
    frame condition #0 (active) {
      n235 = Variant To Data(type=refnum<k24> refnum ("ILabVIEW In"), Variant=w529) -> (data=w528:refnum<k24>)  [unwired: 1 in, 1 out]
      n236 = call "Std_Bus_Close_System.vi"("ILabVIEW In"=w528) -> ("error out"=w530:errorcluster)  [unwired: 1 in, 17 out]
    }
    frame condition #1 {
    }
  }
  n237 = Unbundle By Name(w5) -> ("Handle"=w2)
  n238 = Unbundle By Name(w4) -> ("Handle"=w1)
  n239 = disable-structure shown="Disabled" {
    frame Disabled {
      (unwired) string[] ["Cookbook Stopped"] ("[user-defined descriptions]")
      w533 = T22 2 items=["no dialog", "OK message", "continue or stop message", "OK message + warnings", "continue/stop + warnings"] ("type of dialog (OK msg:1)")
      n240 = call <vilib>:"General Error Handler.vi"("[user-defined codes]"=i32[] [5000], "type of dialog (OK msg:1)"=w533) -> ("[user-defined descriptions]"=w535:string[])  [unwired: 8 in, 5 out]
      n241 = One Button Dialog(message="Please Enter \nAn Observer\nAnd A Comment") -> ()  [unwired: 1 in, 1 out]
    }
    frame Enabled {
    }
  }
  n242 = call "SCMP Andor Neo Close.vi"("error in (no error)"=w27, 10:w1, "Andor Neo"=w2) -> ("error out"=w30:errorcluster)  [unwired: 8 in]
  n243 = Merge Errors(w30, w25, w26) -> (w19:errorcluster)
  "Last Error" <- w19
  n244 = Unbundle By Name(w19) -> ("status"=w10:bool)
  n245 = And(x=FALSE, y=w10) -> (x .and. y?=→"Program":bool)
